vi "LabVIEW Task Manager.vi"() -> ()   [LabVIEW 2013, in "LVTM.lvlib"]
doc: "A debugging tool for use during LabVIEW development. Displays detailed information on all VIs in memory, belonging to a selected project/target. Allows for interacting with single or multiple selected VIs at a time; such as Open/Close their FP or BD, toggle execution highlighting, Pause/Resume/TogglePause their execution state, and more. Aborting selected VIs is also available for top-level VIs, but not for statically called SubVIs [reserved, waiting to run], nor most clones).\n\nNote: \"Refresh\" is not the same as \"Update\". The Update Speed determines how often State, Paused?, Hilite?, and Data Size properties are updated, plus removes items that are no longer in memory. A Refresh operation will repopulate the table with items which have come into memory since the last Refresh operation. A Refresh operation can be manually invoked from the View menu or by pressing F5, and is automatically invoked when any of the item Filter (include/exclude) options are toggled."
uses:
  LVTM.lvlib
  Controls_LVTM/View.ctl
  Controls_LVTM/SharedDataDVR.ctl
  Plugin/LVTM_Plugin.lvclass
  Controls_LVTM/LVTM_Config_Info.ctl
  TCP_Server/TCP_Server.lvclass
  <vilib>/GPower/Error/SubVIs/Filter/Error_FilterMulti.vi
  VIs_LVTM/FindName Task_Manager Library/FindName Task_Manager.lvlib
  DiscoverCommonTypeDefCallers.lvlib
  <userlib>/_SmartBalloon/Engine/Engine.lvclass
  HelpAbout_rha/RHA.lvlib
panel:
  in  "Search Clones Up To":i32=100 caption="Max Clones" min=0 step=1
  in  "Toggle Pause":bool
  in  "Pause":bool
  in  "Resume":bool
  in  "Do Not Highlight Execution":bool
  in  "Highlight Execution":bool
  in  "Close Front Panel":bool
  in  "Close Block Diagram":bool
  in  "Open Front Panel":bool
  in  "Open Block Diagram":bool
  in  "Abort":bool
  in  "App Instance:":u16(ring) items=["Default Application Instance", "Task Manager.lvproj:My Computer"]
  in  "View":T1
  out "NameFilterIsActive":bool
  out "FindIsActive":bool
  in  "error in":errorcluster
  in  "Refresh":bool
  in  "Data Tree":string[](tree)=["Get File Extension.vi"]
  out "Active Filters":string
  in  "Pause Source":string
  in  "Initialize":bool
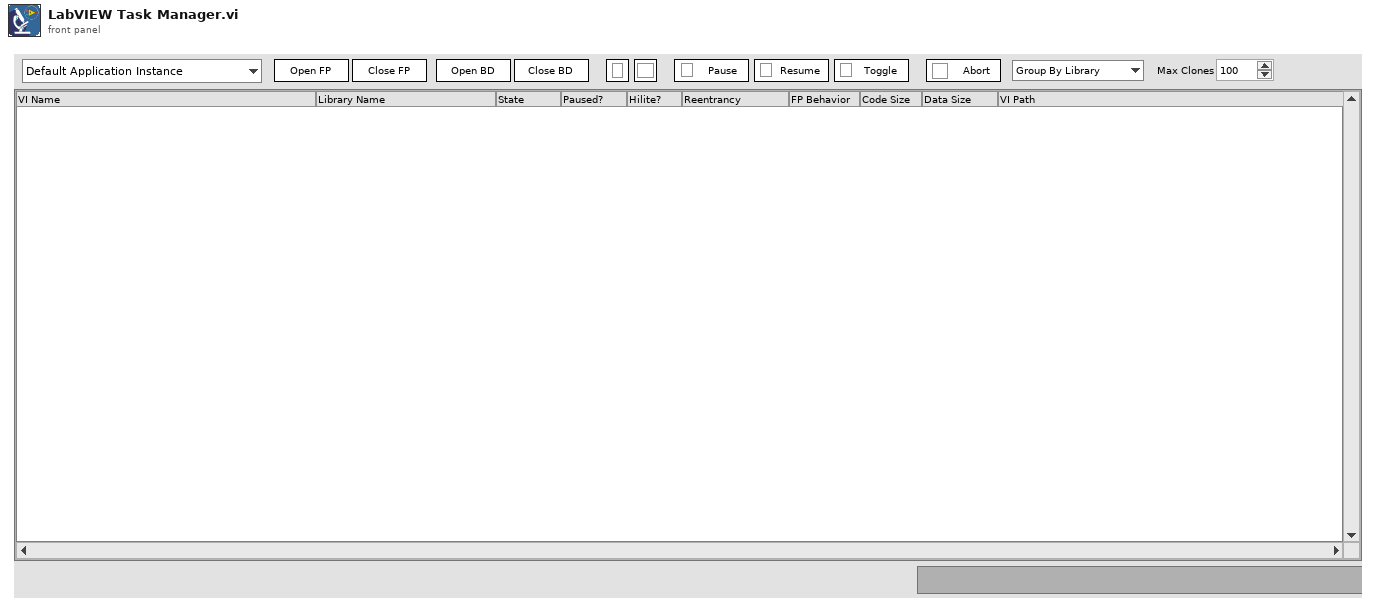
[diagram p1: front panel]
types:
  T1 = typedef "LVTM.lvlib/View.ctl" = enum16{"Group By Library", "Group By Folder", "Flat List"}
  T2 = typedef "LVTM.lvlib/LVTM_Config_Info.ctl" = cluster{"Data Tree Ref":refnum<vi>, "FP Ref":refnum<vi>, "Column Data Type":enum16{"String", "Numeric"}[], "Search Clones Up To":i32, "SortOptions":cluster{"Col.pri":i32, "RevDir.pri":bool, "Col.sec":i32, "RevDir.sec":bool}, "Group/Flat (0:group)":bool, "CollapsedNodes":string[], "Show/Hide Cols":bool[], "Filtered Paths":path[], "View":T1, "File Extension Filters":string[], "Filter Global VIs":bool, "Shared":refnum<data-value>, "Active Filters":refnum<vi>, "Refresh Rate (ms)":i32}
  T3 = cluster{"Shared":refnum<data-value>, "Plugins":refnum<class "LVTM_Plugin.lvclass">[], "UIConfig":T2}
  T4 = typedef "LVTM.lvlib/RequestEvents.ctl" = cluster{"Pause":refnum<user-event>, "Handle Error":refnum<user-event>, "Update Items":refnum<user-event>}
  T5 = typedef "LVTM.lvlib/SharedDataDVR.ctl" = cluster{"App":refnum<vi>, "VIs":string[]}
  T6 = enum16{"Share clones between instances", "Preallocate clone for each instance"}
  T7 = enum32{"Bad", "Idle", "Run top level", "Running"}
  T8 = typedef "LVPoint32TypeDef.ctl" = cluster{"Horizontal":i32, "Vertical":i32}
  T9 = enum32{"Invalid", "Standard", "Closed", "Hidden", "Minimized", "Maximized"}
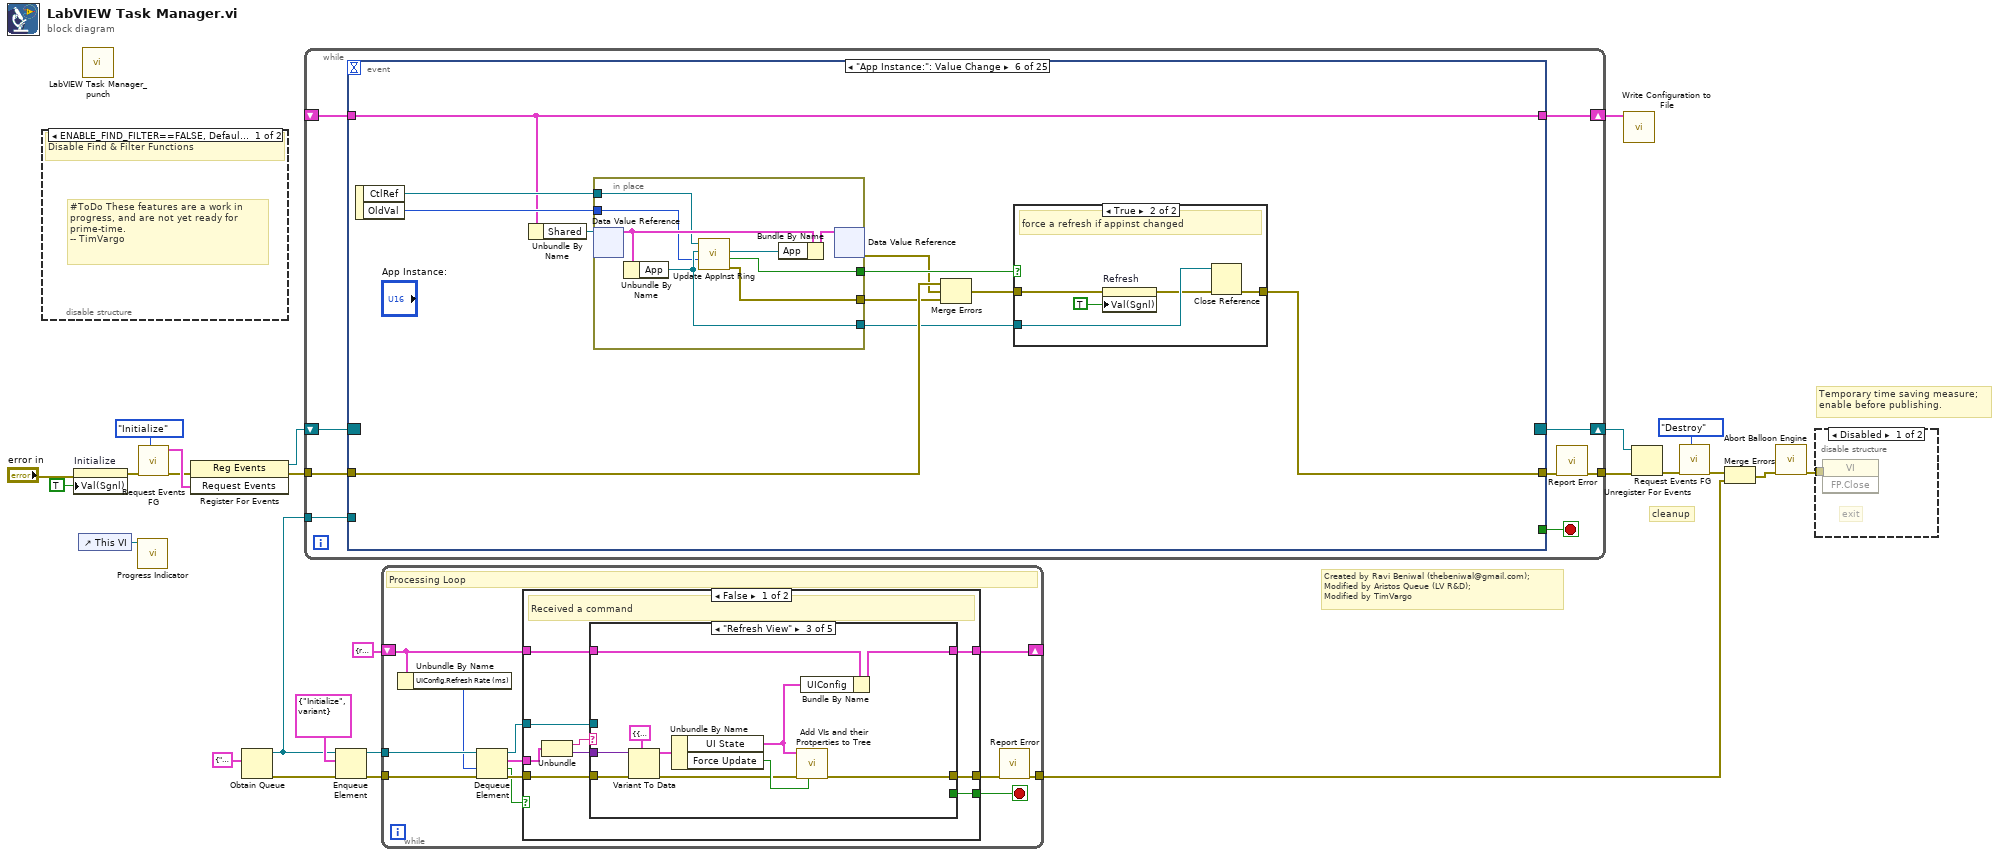
[diagram p0: block diagram]
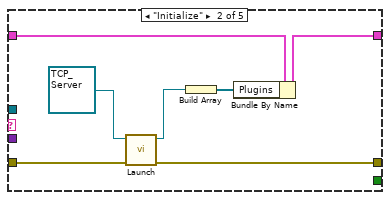
[diagram p4: hidden frame]
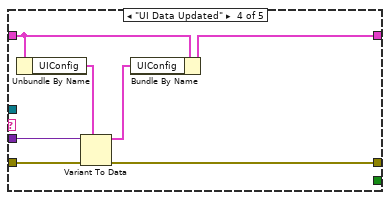
[diagram p5: hidden frame]
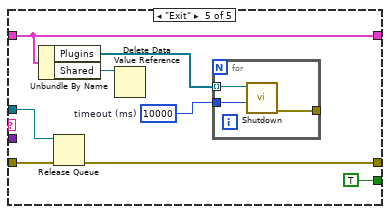
[diagram p6: hidden frame]
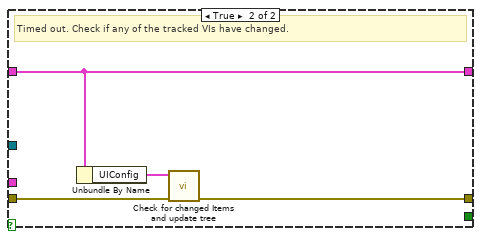
[diagram p7: hidden frame]
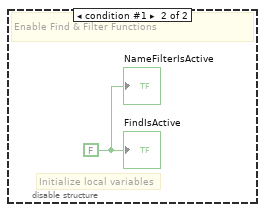
[diagram p8: hidden frame]
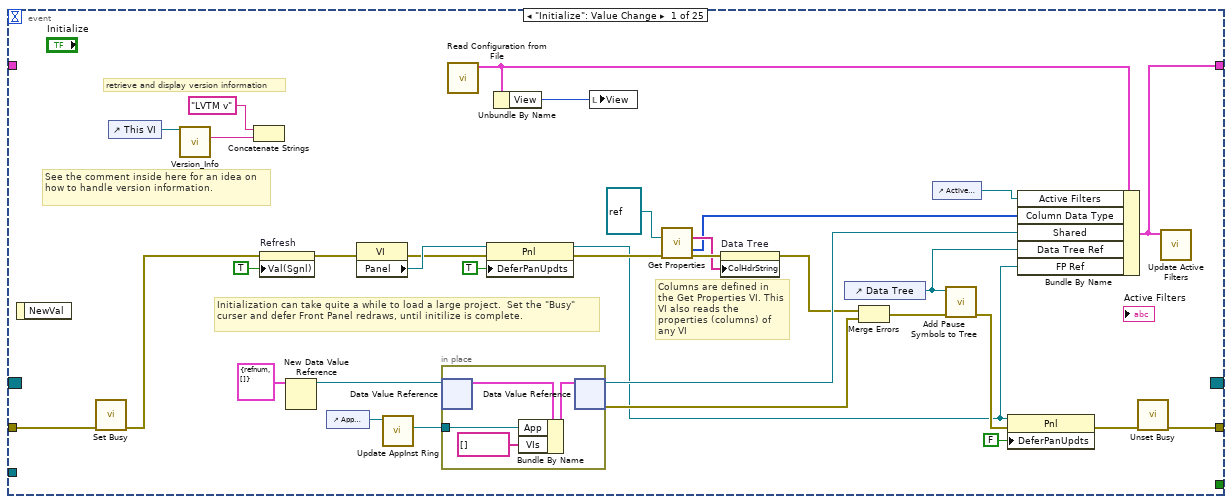
[diagram p9: hidden frame]
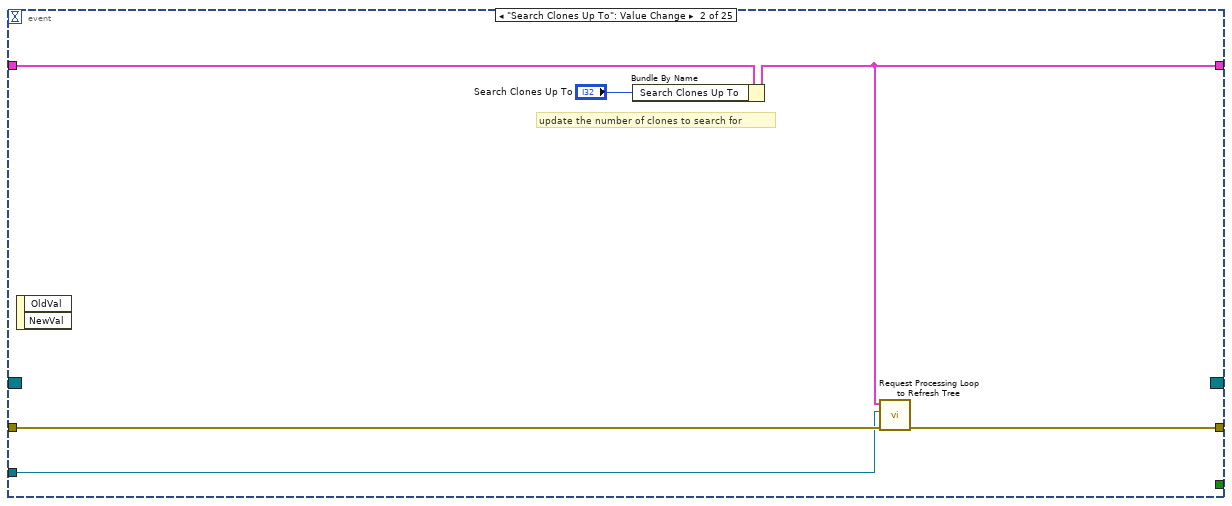
[diagram p10: hidden frame]
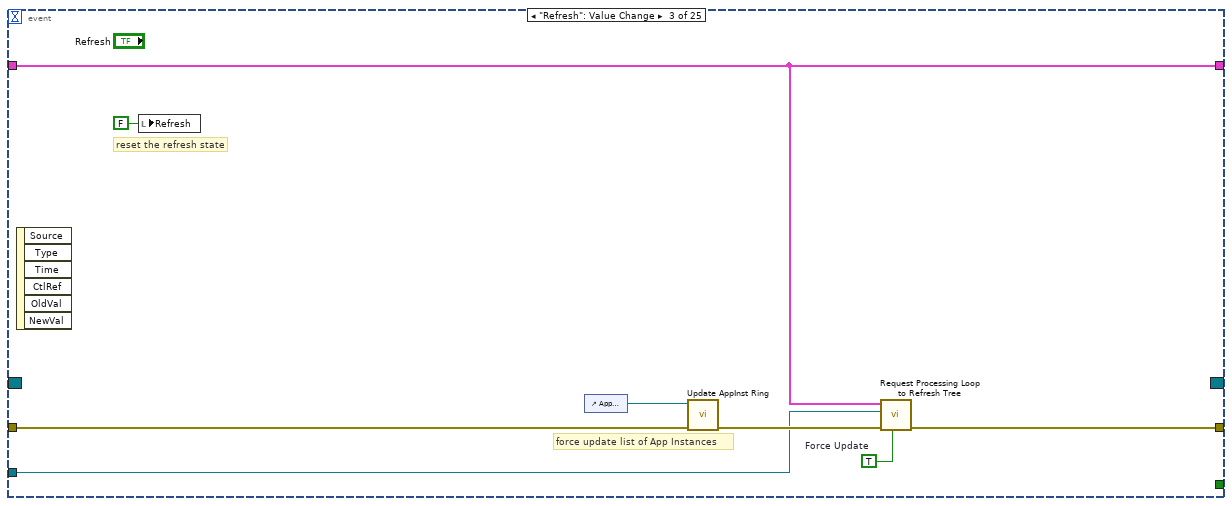
[diagram p11: hidden frame]
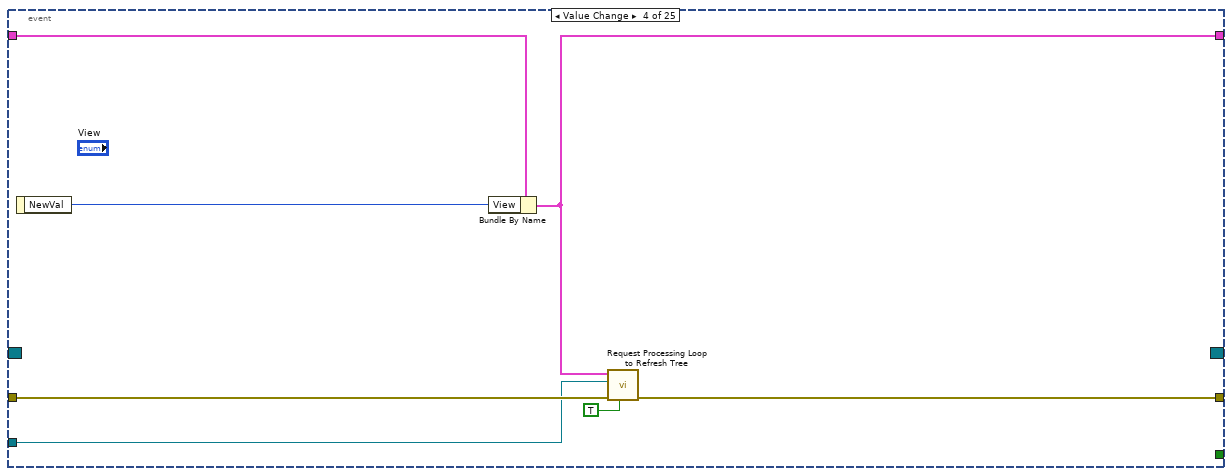
[diagram p12: hidden frame]
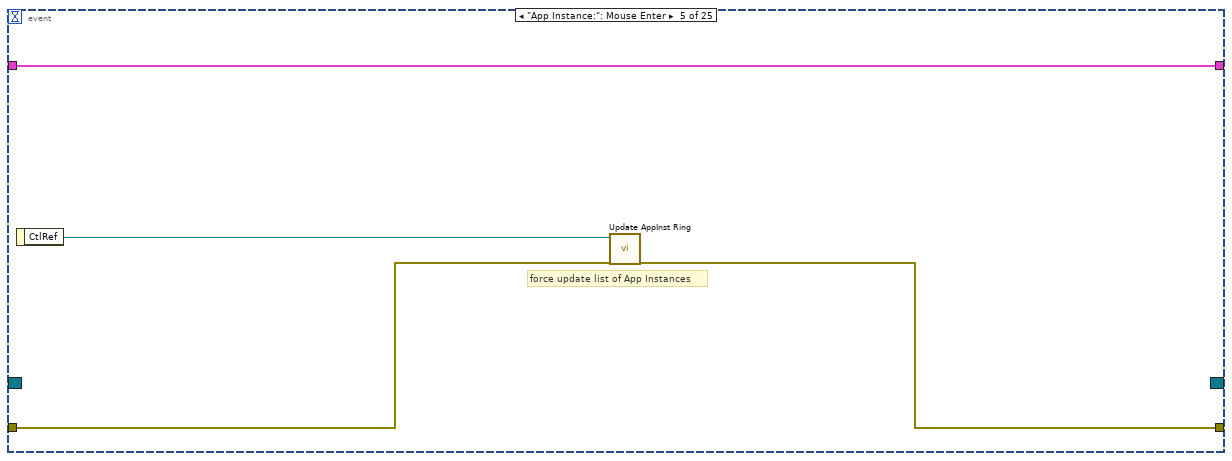
[diagram p13: hidden frame]
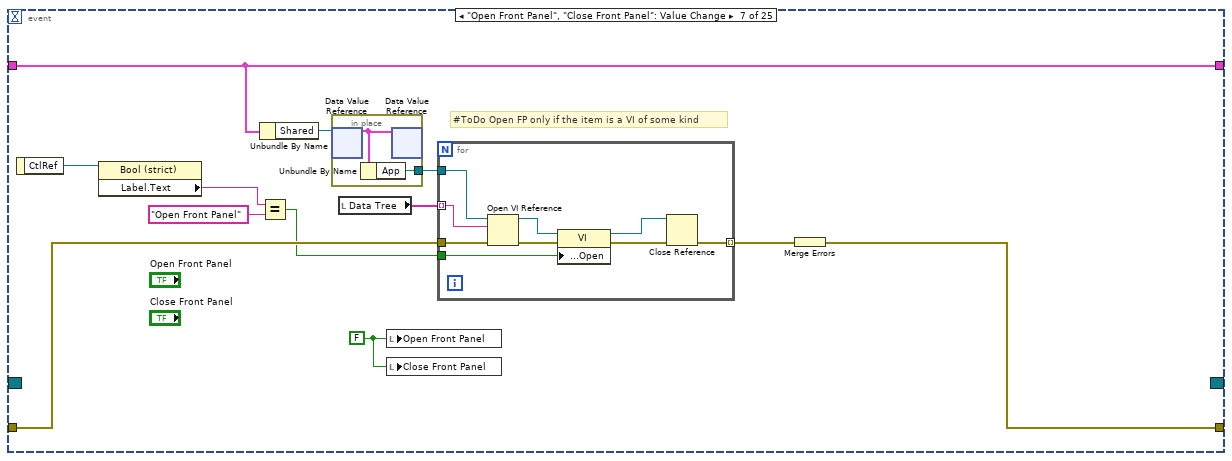
[diagram p15: hidden frame]
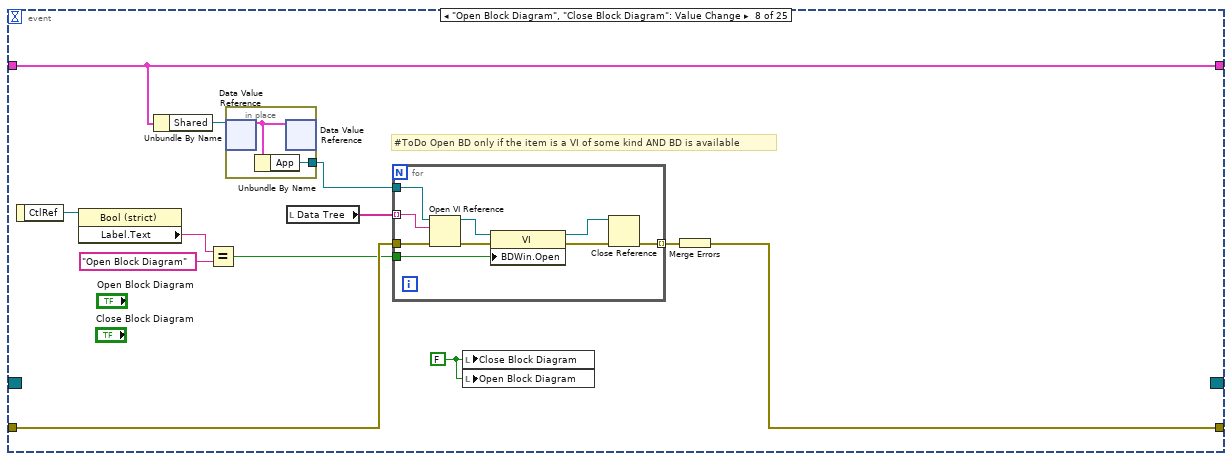
[diagram p16: hidden frame]
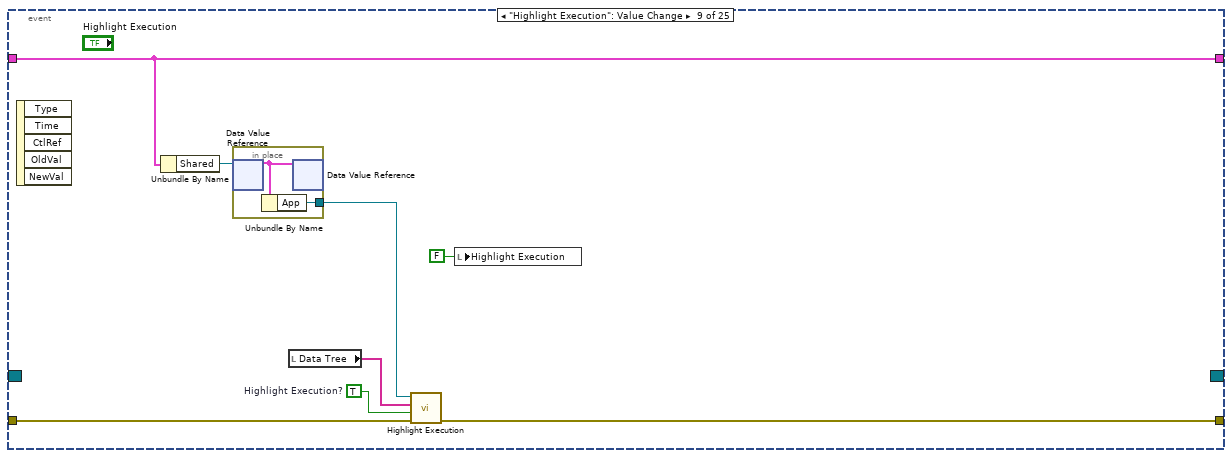
[diagram p17: hidden frame]
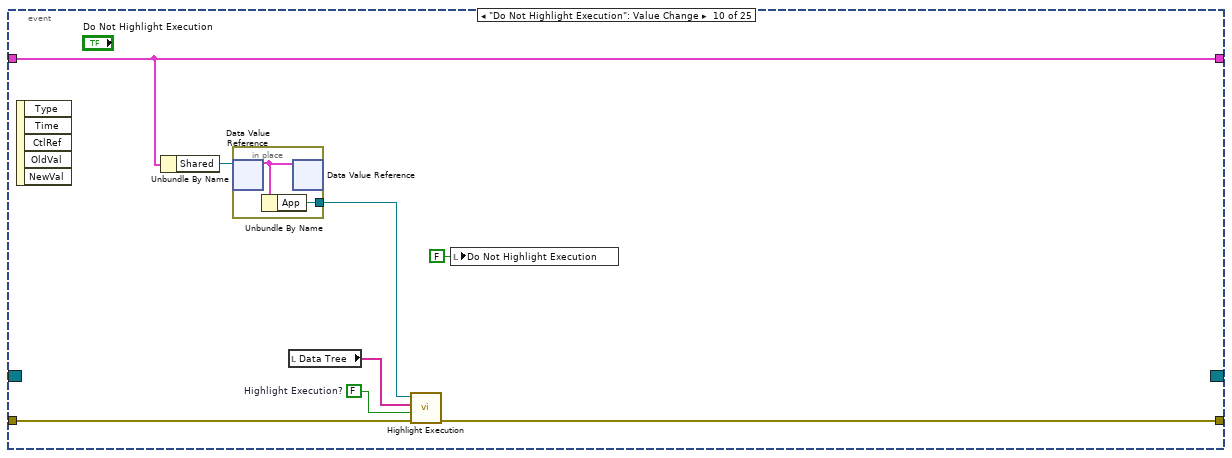
[diagram p18: hidden frame]
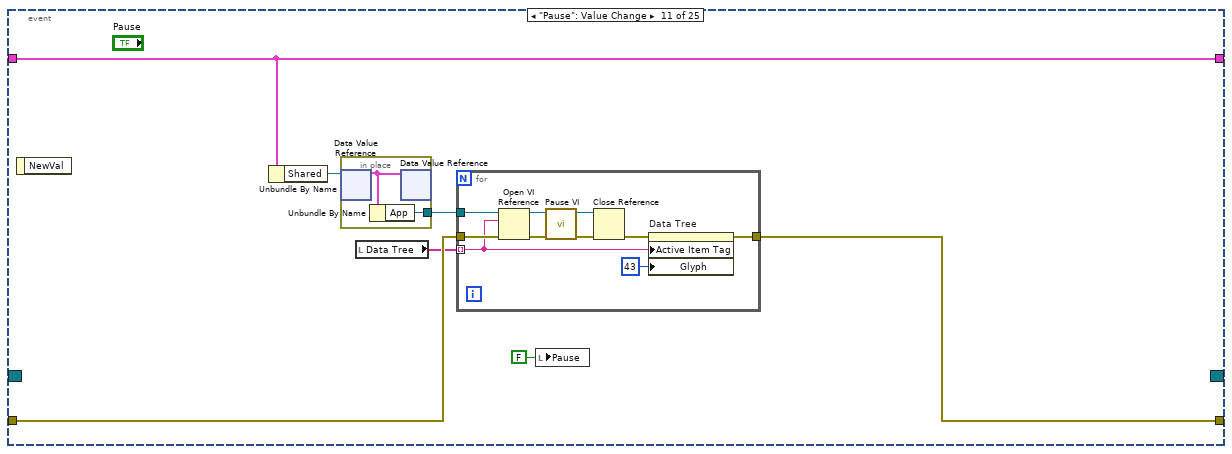
[diagram p19: hidden frame]
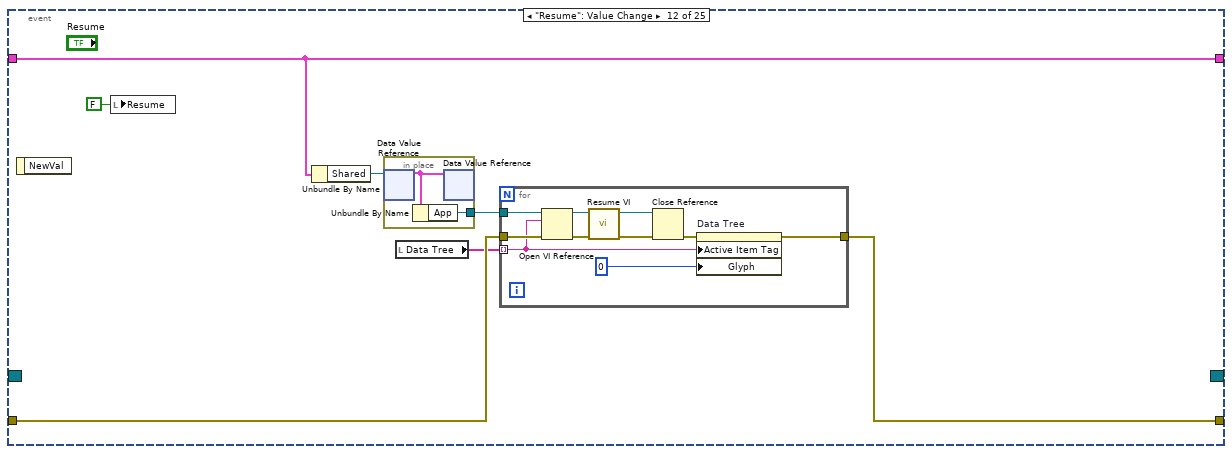
[diagram p20: hidden frame]
diagram:
  # "Temporary time saving measure;\nenable before publishing."
  # "cleanup"
  # "Created by Ravi Beniwal (thebeniwal@gmail.com);\nModified by Aristos Queue (LV R&D);\nModified by TimVargo"
  n1 = disable-structure shown="ENABLE_FIND_FILTER==FALSE, Default" {
    frame condition #0 (active) {
      # "#ToDo These features are a work in progress, and are not yet ready for prime-time.\n-- TimVargo"
      # "Disable Find & Filter Functions"
    }
    frame condition #1 {
      w26 = FALSE ("FindIsActive")
      # "Initialize local variables"
      # "Enable Find & Filter Functions"
      "FindIsActive" <- w26
      "NameFilterIsActive" <- w26
    }
  }
  n2 = property on="Initialize" class="Bool (strict)"(error in="error in", "Val(Sgnl)"=TRUE ("Value (Signaling)")) -> (error out=w16:errorcluster)  [unwired: 1 in, 1 out]
  n3 = control-ref of="This VI"() -> (w9:refnum<vi>)
  n4 = call "LabVIEW Task Manager_punch.vi"() -> ()  [unwired: 12 in]
  n5 = call "Progress Indicator.vi"("Main VI Ref"=w9) -> ()  [unwired: 11 in]
  n6 = call "Request Events FG.vi"("Action (Get)"=enum16{"Initialize", "Get", "Destroy"}."Initialize" ("Action"), "error in"=w16) -> ("error out"=w15:errorcluster, "Request Events"=w18:T4)  [unwired: 8 in]
  n7 = register-events(error in=w15, w18) -> (reference out=w23:refnum<event-registration>, error out=w22:errorcluster)  [unwired: 1 in]
  n8 = Obtain Queue(element data type=cluster{"Command":string, "Data":variant} {"Command"="", "Data"=variant}) -> (queue out=w7:refnum<queue>, error out=w5:errorcluster)  [unwired: 4 in, 1 out]
  n9 = while {
    shift-right: [w27] -> w10
    shift-left: _ -> [w34]
    shift-right: [w33] -> w24
    shift-left: w23 -> [w32]
    tunnel: w22 -> [w31]
    tunnel: [w29] -> w21
    tunnel: w7 -> [w28]
    stop <- w35 stop-if-true
    n10 = event shown="[5] \"App Instance:\": Value Change" {
      selector: w32 -> [_ _ _ _ _ _ _ _ _ _ _ _ _ _ _ _ _ _ _ _ _ _ _ _ _]
      dyn-events: [_ _ _ _ _ _ _ _ _ _ _ _ _ _ _ _ _ _ _ _ _ _ _ _ _] -> w33
      timeout: _ -> [_ _ _ _ _ _ _ _ _ _ _ _ _ _ _ _ _ _ _ _ _ _ _ _ _]
      tunnel: [_ _ _ _ _ _ _ _ _ _ _ _ _ _ _ _ _ _ w457 TRUE ("stop") _ _ w519 _ _] -> w35
      tunnel: w34 -> [_ w78 w85 w93 w97 w101 w125 w148 w172 w182 w195 w209 w231 w253 w294 w301 w357 w397 w464 w470 w481 w483 w515 w718 w751]
      tunnel: [w38 w74 w85 w88 w97 w101 w125 w148 w172 w182 w195 w209 w231 w253 w294 w302 w357 w397 w464 w470 w481 w483 w514 w718 w749] -> w27
      tunnel: w31 -> [w61 w77 w84 w92 w95 w108 w134 w157 w176 w186 w194 w214 w228 w256 w291 w300 w364 w402 w456 w472 _ w492 w517 w719 w752]
      tunnel: [w59 w76 w82 w91 w94 w107 w127 w150 w175 w185 w193 w213 w230 w255 w290 w296 w362 w401 w456 w469 _ w487 w516 w717 w750] -> w30
      tunnel: w28 -> [_ w73 w81 w87 _ _ _ _ _ _ _ _ _ _ _ w295 _ _ w455 w471 _ _ w513 _ _]
      event "Initialize": Value Change {
        # "See the comment inside here for an idea on how to handle version information."
        # "retrieve and display version information"
        # "Initialization can take quite a while to load a large project.  Set the \"Busy\" curser and defer Front Panel redraws, until initilize is complete."
        # "Columns are defined in the Get Properties VI. This VI also reads the properties (columns) of any VI"
        n11 = event-data() -> ()  [unwired: 2 out]
        n12 = call <vilib>:"Set Busy.vi"("error in (no error)"=w61) -> ("error out"=w54:errorcluster)  [unwired: 9 in, 1 out]
        n13 = control-ref of="This VI"() -> (w50:refnum<vi>)
        n14 = call "Version_Info.vi"("Generic VI Reference"=w50) -> ("FileVersion_Str"=w49:string)  [unwired: 8 in, 2 out]
        n15 = Concatenate Strings("LVTM v" ("string"), w49) -> ()  [unwired: 1 out]
        n16 = property on="Refresh" class="Bool (strict)"(error in=w54, "Val(Sgnl)"=TRUE ("Value (Signaling)")) -> (error out=w66:errorcluster)  [unwired: 1 in, 1 out]
        n17 = New Data Value Reference(data value=T5 {"App"=refnum, "VIs"=[]}) -> (data value reference=w36:refnum<data-value>)  [unwired: 1 in, 1 out]
        n18 = control-ref of="App Instance:"() -> (w67:refnum<vi>)
        n19 = property class="VI"(error in=w66) -> (error out=w52:errorcluster, "Panel"=w53:refnum<vi>)  [unwired: 1 in, 1 out]
        n20 = call "Update AppInst Ring.vi"("Ring in"=w67) -> ("AppInst out"=w47:refnum<vi>)  [unwired: 8 in, 2 out]
        n21 = in-place {
          in-place-border: w47 -> [w69]
          n22 = in-place-dvr #1(w36) -> (w72:T5)  [unwired: 1 out]
          n23 = Bundle By Name(cluster=w72, "App"=w69, "VIs"=string[] []) -> (w71:T5)
          n24 = in-place-dvr #1(w71) -> (w46:refnum<data-value>, w43:errorcluster)
        }
        n25 = call "Read Configuration from File.vi"() -> ("Configuration"=w41:T2)  [unwired: 10 in, 1 out]
        n26 = property class="Pnl"(reference=w53, error in=w52, "DeferPanUpdts"=TRUE ("Defer Panel Updates")) -> (reference out=w40:refnum<vi>, error out=w51:errorcluster)
        n27 = Unbundle By Name(w41) -> ("View"=w42:T1)
        n28 = local write "View"(w42) -> ()
        n29 = call "Get Properties.vi"("AppInst"=refnum<vi> refnum, "error in"=w51) -> ("Column Labels"=w64:string[], "Column Data Type"=w60:enum16{"String", "Numeric"}[], "error out"=w65:errorcluster)  [unwired: 4 in, 7 out]
        n30 = property on="Data Tree" class="Tree (strict)"(error in=w65, "ColHdrString"=w64) -> (error out=w45:errorcluster)  [unwired: 1 in, 1 out]
        n31 = control-ref of="Data Tree"() -> (w62:refnum<vi>)
        n32 = Merge Errors(w45, w43) -> (w44:errorcluster)
        n33 = control-ref of="Active Filters"() -> (w39:refnum<vi>)
        n34 = call "Add Pause Symbols to Tree.vi"("error in"=w44, "Data Tree Ref"=w62) -> ("error out"=w56:errorcluster)  [unwired: 9 in]
        n35 = property class="Pnl"(reference=w40, error in=w56, "DeferPanUpdts"=FALSE ("Defer Panel Updates")) -> (error out=w55:errorcluster)  [unwired: 1 out]
        n36 = Bundle By Name(cluster=w41, "Active Filters"=w39, "Column Data Type"=w60, "Shared"=w46, "Data Tree Ref"=w62, "FP Ref"=w40) -> (w38:T2)
        n37 = call <vilib>:"Unset Busy.vi"("error in (no error)"=w55) -> ("error out"=w59:errorcluster)  [unwired: 10 in]
        n38 = call "Update Active Filters.vi"("Configuration"=w38) -> ()  [unwired: 10 in, 1 out]
      }
      event "Search Clones Up To": Value Change {
        # "update the number of clones to search for"
        n39 = event-data() -> ()  [unwired: 3 out]
        n40 = Bundle By Name(cluster=w78, "Search Clones Up To"="Search Clones Up To") -> (w74:T2)
        n41 = call "Request Processing Loop to Refresh Tree.vi"("error in (no error)"=w77, "Queue in"=w73, "ConfigInfo in"=w74) -> ("error out"=w76:errorcluster)  [unwired: 8 in]
      }
      event "Refresh": Value Change {
        w79 = TRUE  # Force Update
        # "reset the refresh state"
        # "force update list of App Instances"
        n42 = event-data() -> ()  [unwired: 7 out]
        n43 = local write "Refresh"(FALSE ("Refresh")) -> ()
        n44 = control-ref of="App Instance:"() -> (w86:refnum<vi>)
        n45 = call "Update AppInst Ring.vi"("error in"=w84, "Ring in"=w86) -> ("error out"=w83:errorcluster)  [unwired: 7 in, 2 out]
        n46 = call "Request Processing Loop to Refresh Tree.vi"("Force Update"=w79, "error in (no error)"=w83, "Queue in"=w81, "ConfigInfo in"=w85) -> ("error out"=w82:errorcluster)  [unwired: 7 in]
      }
      event Value Change {
        n47 = event-data() -> ("NewVal"=w90:T1)  [unwired: 1 out]
        n48 = Bundle By Name(cluster=w93, "View"=w90) -> (w88:T2)
        n49 = call "Request Processing Loop to Refresh Tree.vi"("Force Update"=TRUE ("Force Tree Update (F)"), "error in (no error)"=w92, "Queue in"=w87, "ConfigInfo in"=w88) -> ("error out"=w91:errorcluster)  [unwired: 7 in]
      }
      event "App Instance:": Mouse Enter {
        # "force update list of App Instances"
        n50 = event-data() -> ("CtlRef"=w96:refnum<vi>)  [unwired: 1 out]
        n51 = call "Update AppInst Ring.vi"("error in"=w95, "Ring in"=w96) -> ("error out"=w94:errorcluster)  [unwired: 7 in, 2 out]
      }
      event "App Instance:": Value Change {
        n52 = event-data() -> ("CtlRef"=w104:refnum<vi>, "OldVal"=w103:u16)  [unwired: 1 out]
        n53 = Unbundle By Name(w101) -> ("Shared"=w106:refnum<data-value>)
        n54 = in-place {
          in-place-border: [w114] -> w105
          in-place-border: w104 -> [w115]
          in-place-border: w103 -> [w113]
          in-place-border: [w110] -> w102
          in-place-border: [w109] -> w98
          n55 = in-place-dvr #2(w106) -> (w116:T5)  [unwired: 1 out]
          n56 = Unbundle By Name(w116) -> ("App"=w114:refnum<vi>)
          n57 = call "Update AppInst Ring.vi"("Old Value"=w113, "AppInst in"=w114, "Ring in"=w115) -> ("error out"=w109:errorcluster, "Selection Changed?"=w110:bool, "AppInst out"=w111:refnum<vi>)  [unwired: 6 in]
          n58 = Bundle By Name(cluster=w116, "App"=w111) -> (w112:T5)
          n59 = in-place-dvr #2(w112) -> (w99:errorcluster)  [unwired: 1 out]
        }
        n60 = Merge Errors(w108, w99, w98) -> (w100:errorcluster)
        n61 = case shown="True" w102 {
          tunnel: w105 -> [_ w121]
          tunnel: w100 -> [w117 w120]
          tunnel: [w117 w118] -> w107
          frame False {
            # "do nothing"
          }
          frame True {
            # "force a refresh if appinst changed"
            n62 = property on="Refresh" class="Bool (strict)"(error in=w120, "Val(Sgnl)"=TRUE ("Value (Signaling)")) -> (error out=w119:errorcluster)  [unwired: 1 in, 1 out]
            n63 = Close Reference(reference=w121, error in (no error)=w119) -> (error out=w118:errorcluster)
          }
        }
      }
      event "Open Front Panel", "Close Front Panel": Value Change {
        w123 = FALSE ("Open Front Panel")
        # "#ToDo Open FP only if the item is a VI of some kind"
        n64 = event-data() -> ("CtlRef"=w131:refnum<vi>)  [unwired: 1 out]
        n65 = property class="Bool (strict)"(reference=w131) -> ("Label.Text"=w129:string)  [unwired: 1 in, 2 out]
        n66 = Unbundle By Name(w125) -> ("Shared"=w126:refnum<data-value>)
        n67 = Equal?(x=w129, y="Open Front Panel") -> (x = y?=w128:bool)
        n68 = in-place {
          in-place-border: [w135] -> w124
          n69 = in-place-dvr #3(w126) -> (w136:T5)  [unwired: 1 out]
          n70 = Unbundle By Name(w136) -> ("App"=w135:refnum<vi>)
          n71 = in-place-dvr #3(w136) -> ()  [unwired: 2 out]
        }
        n72 = local read "Data Tree"() -> (w132:string[])
        n73 = local write "Open Front Panel"(w123) -> ()
        n74 = local write "Close Front Panel"(w123) -> ()
        n75 = for {
          tunnel: [w145] -> w133 mode=indexing
          tunnel: w134 -> [w144]
          tunnel: w132 -> [w143] mode=indexing
          tunnel: w124 -> [w138]
          tunnel: w128 -> [w137]
          n76 = Open VI Reference(application reference (local)=w138, vi path=w143, error in (no error)=w144) -> (vi reference=w141:refnum<vi>, error out=w142:errorcluster)  [unwired: 3 out]
          n77 = property class="VI"(reference=w141, error in=w142, "Front Panel.Open"=w137) -> (reference out=w140:refnum<vi>, error out=w139:errorcluster)
          n78 = Close Reference(reference=w140, error in (no error)=w139) -> (error out=w145:errorcluster)
        }
        n79 = Merge Errors(w133) -> (w127:errorcluster)
      }
      event "Open Block Diagram", "Close Block Diagram": Value Change {
        w146 = FALSE ("Close Block Diagram")
        # "#ToDo Open BD only if the item is a VI of some kind AND BD is available"
        n80 = event-data() -> ("CtlRef"=w152:refnum<vi>)  [unwired: 1 out]
        n81 = property class="Bool (strict)"(reference=w152) -> ("Label.Text"=w153:string)  [unwired: 1 in, 2 out]
        n82 = Unbundle By Name(w148) -> ("Shared"=w149:refnum<data-value>)
        n83 = Equal?(x=w153, y="Open Block Diagram") -> (x = y?=w151:bool)
        n84 = in-place {
          in-place-border: [w158] -> w147
          n85 = in-place-dvr #4(w149) -> (w159:T5)  [unwired: 1 out]
          n86 = Unbundle By Name(w159) -> ("App"=w158:refnum<vi>)
          n87 = in-place-dvr #4(w159) -> ()  [unwired: 2 out]
        }
        n88 = local read "Data Tree"() -> (w155:string[])
        n89 = for {
          tunnel: [w168] -> w156 mode=indexing
          tunnel: w157 -> [w167]
          tunnel: w155 -> [w166] mode=indexing
          tunnel: w147 -> [w161]
          tunnel: w151 -> [w160]
          n90 = Open VI Reference(application reference (local)=w161, vi path=w166, error in (no error)=w167) -> (vi reference=w164:refnum<vi>, error out=w165:errorcluster)  [unwired: 3 out]
          n91 = property class="VI"(reference=w164, error in=w165, "BDWin.Open"=w160) -> (reference out=w163:refnum<vi>, error out=w162:errorcluster)
          n92 = Close Reference(reference=w163, error in (no error)=w162) -> (error out=w168:errorcluster)
        }
        n93 = local write "Close Block Diagram"(w146) -> ()
        n94 = local write "Open Block Diagram"(w146) -> ()
        n95 = Merge Errors(w156) -> (w150:errorcluster)
      }
      event "Highlight Execution": Value Change {
        w169 = TRUE  # Highlight Execution?
        n96 = event-data() -> ()  [unwired: 6 out]
        n97 = Unbundle By Name(w172) -> ("Shared"=w173:refnum<data-value>)
        n98 = in-place {
          in-place-border: [w177] -> w171
          n99 = in-place-dvr #5(w173) -> (w178:T5)  [unwired: 1 out]
          n100 = Unbundle By Name(w178) -> ("App"=w177:refnum<vi>)
          n101 = in-place-dvr #5(w178) -> ()  [unwired: 2 out]
        }
        n102 = local read "Data Tree"() -> (w174:string[])
        n103 = call "Highlight Execution.vi"("error in (no error)"=w176, "Highlight Execution?"=w169, "VIs"=w174, "Application in"=w171) -> ("error out"=w175:errorcluster)  [unwired: 7 in]
        n104 = local write "Highlight Execution"(FALSE ("Toggle ExecHilite")) -> ()
      }
      event "Do Not Highlight Execution": Value Change {
        w179 = FALSE  # Highlight Execution?
        n105 = event-data() -> ()  [unwired: 6 out]
        n106 = Unbundle By Name(w182) -> ("Shared"=w183:refnum<data-value>)
        n107 = in-place {
          in-place-border: [w187] -> w181
          n108 = in-place-dvr #6(w183) -> (w188:T5)  [unwired: 1 out]
          n109 = Unbundle By Name(w188) -> ("App"=w187:refnum<vi>)
          n110 = in-place-dvr #6(w188) -> ()  [unwired: 2 out]
        }
        n111 = local read "Data Tree"() -> (w184:string[])
        n112 = call "Highlight Execution.vi"("error in (no error)"=w186, "Highlight Execution?"=w179, "VIs"=w184, "Application in"=w181) -> ("error out"=w185:errorcluster)  [unwired: 7 in]
        n113 = local write "Do Not Highlight Execution"(FALSE ("Toggle ExecHilite")) -> ()
      }
      event "Pause": Value Change {
        n114 = event-data() -> ()  [unwired: 2 out]
        n115 = Unbundle By Name(w195) -> ("Shared"=w191:refnum<data-value>)
        n116 = in-place {
          in-place-border: [w196] -> w190
          n117 = in-place-dvr #7(w191) -> (w197:T5)  [unwired: 1 out]
          n118 = Unbundle By Name(w197) -> ("App"=w196:refnum<vi>)
          n119 = in-place-dvr #7(w197) -> ()  [unwired: 2 out]
        }
        n120 = local read "Data Tree"() -> (w192:string[])
        n121 = for {
          tunnel: w192 -> [w200] mode=indexing
          tunnel: w194 -> [w203]
          tunnel: [w201] -> w193
          tunnel: w190 -> [w198]
          n122 = Open VI Reference(application reference (local)=w198, vi path=w200, error in (no error)=w203) -> (vi reference=w206:refnum<vi>, error out=w207:errorcluster)  [unwired: 3 out]
          n123 = call "Pause VI.vi"("error in (no error)"=w207, "VI in"=w206) -> ("error out"=w204:errorcluster, "VI out"=w205:refnum<vi>)  [unwired: 8 in]
          n124 = Close Reference(reference=w205, error in (no error)=w204) -> (error out=w202:errorcluster)
          n125 = property on="Data Tree" class="Tree (strict)"(error in=w202, "Active Item Tag"=w200, "Glyph"=43 ("Active Item:Symbol Index")) -> (error out=w201:errorcluster)  [unwired: 1 in, 1 out]
        }
        n126 = local write "Pause"(FALSE ("Pause")) -> ()
      }
      event "Resume": Value Change {
        n127 = event-data() -> ()  [unwired: 2 out]
        n128 = local write "Resume"(FALSE ("Resume")) -> ()
        n129 = Unbundle By Name(w209) -> ("Shared"=w210:refnum<data-value>)
        n130 = in-place {
          in-place-border: [w215] -> w208
          n131 = in-place-dvr #8(w210) -> (w216:T5)  [unwired: 1 out]
          n132 = Unbundle By Name(w216) -> ("App"=w215:refnum<vi>)
          n133 = in-place-dvr #8(w216) -> ()  [unwired: 2 out]
        }
        n134 = local read "Data Tree"() -> (w212:string[])
        n135 = for {
          tunnel: w212 -> [w218] mode=indexing
          tunnel: w214 -> [w222]
          tunnel: [w219] -> w213
          tunnel: w208 -> [w217]
          n136 = Open VI Reference(application reference (local)=w217, vi path=w218, error in (no error)=w222) -> (vi reference=w225:refnum<vi>, error out=w226:errorcluster)  [unwired: 3 out]
          n137 = call "Resume VI.vi"("error in (no error)"=w226, "VI in"=w225) -> ("error out"=w223:errorcluster, "VI out"=w224:refnum<vi>)  [unwired: 8 in]
          n138 = Close Reference(reference=w224, error in (no error)=w223) -> (error out=w220:errorcluster)
          n139 = property on="Data Tree" class="Tree (strict)"(error in=w220, "Active Item Tag"=w218, "Glyph"=0 ("Active Item:Symbol Index")) -> (error out=w219:errorcluster)  [unwired: 1 in, 1 out]
        }
      }
      event "Toggle Pause": Value Change {
        n140 = event-data() -> ()  [unwired: 2 out]
        n141 = local write "Toggle Pause"(FALSE ("Resume")) -> ()
        n142 = Unbundle By Name(w231) -> ("Shared"=w232:refnum<data-value>)
        n143 = in-place {
          in-place-border: [w249] -> w229
          n144 = in-place-dvr #9(w232) -> (w250:T5)  [unwired: 1 out]
          n145 = Unbundle By Name(w250) -> ("App"=w249:refnum<vi>)
          n146 = in-place-dvr #9(w250) -> ()  [unwired: 2 out]
        }
        n147 = local read "Data Tree"() -> (w227:string[])
        n148 = for {
          tunnel: w227 -> [w245] mode=indexing
          tunnel: w228 -> [w248]
          tunnel: [w246] -> w230
          tunnel: w229 -> [w244]
          # "Despite the method name, this\ntoggles Pause/Resume."
          n149 = Open VI Reference(application reference (local)=w244, vi path=w245, error in (no error)=w248) -> (vi reference=w242:refnum<vi>, error out=w243:errorcluster)  [unwired: 3 out]
          n150 = invoke class="VI" method="PauseVI"(reference=w242, error in=w243) -> (reference out=w241:refnum<vi>, error out=w240:errorcluster)  [unwired: 1 in, 1 out]
          n151 = property class="VI"(reference=w241, error in=w240) -> (reference out=w238:refnum<vi>, error out=w239:errorcluster, "Is VI Paused?"=w237:bool)
          n152 = Close Reference(reference=w238, error in (no error)=w239) -> (error out=w247:errorcluster)
          n153 = Select(t=43, s=w237, f=0 ("Active Item:Symbol Index")) -> (s? t:f=w234:i32)
          n154 = property on="Data Tree" class="Tree (strict)"(error in=w247, "Active Item Tag"=w245, "Glyph"=w234) -> (error out=w246:errorcluster)  [unwired: 1 in, 1 out]
        }
      }
      event "Abort": Value Change {
        # "Only VIs running at top level may be aborted."
        # "#ToDo this is where the string 'error' was being placed into the 'library name' column (left of the 'State' column).  This is fixed for now by changing hardwired column number from 1 to 2, but the column number will later need logic to calculate the correct column, once the flat (non-grouped) option is implemented, which will hide the 'library name' column."
        n155 = event-data() -> ()  [unwired: 2 out]
        n156 = Unbundle By Name(w253) -> ("Shared"=w254:refnum<data-value>)
        n157 = local write "Abort"(FALSE ("Abort")) -> ()
        n158 = in-place {
          in-place-border: [w258] -> w252
          n159 = in-place-dvr #10(w254) -> (w259:T5)  [unwired: 1 out]
          n160 = Unbundle By Name(w259) -> ("App"=w258:refnum<vi>)
          n161 = in-place-dvr #10(w259) -> ()  [unwired: 2 out]
        }
        n162 = for {
          tunnel: [w268] -> w255
          tunnel: "Data Tree" -> [w267] mode=indexing
          tunnel: w252 -> [w266]
          tunnel: w256 -> [w265]
          n163 = Open VI Reference(application reference (local)=w266, vi path=w267, error in (no error)=w265) -> (vi reference=w262:refnum<vi>, error out=w264:errorcluster)  [unwired: 3 out]
          n164 = property class="VI"(reference=w262, error in=w264) -> (reference out=w261:refnum<vi>, error out=w263:errorcluster, "Exec.State"=w260:T7)
          n165 = case shown="\"Run top level\"" w260 {
            tunnel: [w269 w281] -> w268
            tunnel: w267 -> [_ w279]
            tunnel: w263 -> [w271 w274]
            tunnel: w261 -> [w270 w273]
            frame "Bad", Default {
              n166 = Close Reference(reference=w270, error in (no error)=w271) -> (error out=w269:errorcluster)
            }
            frame "Run top level" {
              n167 = invoke class="VI" method="Abort VI"(reference=w273, error in=w274) -> (reference out=w283:refnum<vi>, error out=w275:errorcluster)  [unwired: 1 in, 1 out]
              n168 = property class="VI"(reference=w283, error in=w275) -> (reference out=w282:refnum<vi>, error out=w277:errorcluster, "Exec.State"=w284:T7)
              n169 = Close Reference(reference=w282, error in (no error)=w277) -> (error out=w272:errorcluster)
              n170 = case shown="No Error" w272 {
                selector: w272 -> [w285 _]
                tunnel: w284 -> [w288 _]
                tunnel: [w287 "Error"] -> w280
                tunnel: [w286 _] -> w276
                frame No Error {
                  n171 = Format Into String(error in=w285, w288) -> (resulting string=w287:string, error out=w286:errorcluster)  [unwired: 2 in]
                }
                frame Error {
                }
              }
              n172 = property on="Data Tree" class="Tree (strict)"(error in=w276, "Active Item Tag"=w279, "ActiveColNum"=2 ("Active Cell:Active Column Number"), "Cell String"=w280) -> (error out=w281:errorcluster)  [unwired: 1 in, 1 out]
            }
          }
        }
      }
      event "Pause Source": Value Change {
        n173 = event-data() -> ("NewVal"=w292:string)  [unwired: 1 out]
        n174 = property on="Data Tree" class="Tree (strict)"(error in=w291, "Active Item Tag"=w292, "Glyph"=44 ("Active Item:Symbol Index")) -> (error out=w290:errorcluster)  [unwired: 1 in, 1 out]
      }
      event "Data Tree": Mouse Down {
        n175 = event-data() -> ("Coords"=w303:T8)  [unwired: 1 out]
        n176 = invoke on="Data Tree" class="Tree (strict)" method="Point To Row Column"(error in=w300, "Point"=w303) -> (error out=w298:errorcluster, "Tag"=w299:string, "Col"=w297:i32)  [unwired: 6 in, 5 out]
        n177 = case shown="\"TREE_COLUMN_HEADERS\"" w299 {
          tunnel: w298 -> [w305 w322]
          tunnel: w297 -> [_ w325]
          tunnel: [w305 w317] -> w296
          tunnel: [w304 w308] -> w302
          tunnel: w301 -> [w304 w330]
          tunnel: w295 -> [_ w307]
          frame Default {
          }
          frame "TREE_COLUMN_HEADERS" {
            n178 = Unbundle By Name(w330) -> ("Data Tree Ref"=w313:refnum<vi>, "SortOptions.RevDir.pri"=w312:bool, "SortOptions.Col.pri"=w311:i32, "SortOptions.RevDir.sec"=w310:bool, "SortOptions.Col.sec"=w309:i32, "Column Data Type"=w326:enum16{"String", "Numeric"}[], "FP Ref"=w320:refnum<vi>)
            n179 = property class="Pnl"(reference=w320, error in=w322, "DeferPanUpdts"=TRUE ("Defer Panel Updates")) -> (reference out=w316:refnum<vi>, error out=w321:errorcluster)
            n180 = Index Array(array=w326, index=w325) -> (element=w324:enum16{"String", "Numeric"})
            n181 = Equal?(x=w311, y=w325) -> (x = y?=w329:bool)
            n182 = case shown="False" w329 {
              tunnel: w312 -> [w342 w352]
              tunnel: [FALSE ("Sorted AZ?") w351] -> w306
              tunnel: w321 -> [w346 w356]
              tunnel: [w345 w356] -> w328
              tunnel: w325 -> [w344 w355]
              tunnel: [w344 w355] -> w327
              tunnel: w311 -> [w343 _]
              tunnel: [w342 w354] -> w315
              tunnel: w311 -> [w341 _]
              tunnel: [w341 w353] -> w314
              tunnel: w310 -> [_ w354]
              tunnel: w309 -> [_ w353]
              frame False {
                # "New col, update secondaries"
                # "Make new sort column header bold\nand previous sort column header NOT bold"
                # "New col clicked, sort Ascending"
                n183 = property on="Data Tree" class="Tree (strict)"(error in=w346, "Active Item Tag"="TREE_COLUMN_HEADERS" ("Active Item:Tag"), "ActiveColNum"=w343, "CellFontBold"=FALSE ("Active Cell:Cell Font:Bold"), "ActiveColNum"=w344, "CellFontBold"=TRUE ("Active Cell:Cell Font:Bold")) -> (error out=w345:errorcluster)  [unwired: 1 in, 1 out]
              }
              frame True {
                # "Same col, maintain secondaries"
                # "Same col clicked, reverse order"
                n184 = Not(x=w352) -> (.not. x?=w351:bool)
              }
            }
            n185 = case shown="\"String\", Default" w324 {
              tunnel: [w335 w339] -> w318
              tunnel: w306 -> [w334 w338]
              tunnel: w328 -> [w333 w340]
              tunnel: w327 -> [w332 w336]
              tunnel: w313 -> [_ w337]
              frame "String", Default {
                n186 = invoke on="Data Tree" class="Tree (strict)" method="Edit Tree Items.Sort Children"(error in=w333, "Sort Column"=w332, "Sort Recursively"=TRUE ("Sort Recursively?"), "Reverse Order"=w334) -> (error out=w335:errorcluster)  [unwired: 4 in, 7 out]
              }
              frame "Numeric" {
                # "This col contains numeric\ndata and needs to be\nsorted suing special tricks\nas Tree:Sort method only\nsupports Alphabetical sorting."
                n187 = call "Sort Tree Items by Numerical order.vi"("Reverse Order?"=w338, "error in"=w340, "Sort Column"=w336, "Data Tree"=w337) -> ("error out"=w339:errorcluster)  [unwired: 7 in]
              }
            }
            n188 = Bundle By Name(cluster=w330, "SortOptions.RevDir.pri"=w306, "SortOptions.Col.pri"=w327, "SortOptions.RevDir.sec"=w315, "SortOptions.Col.sec"=w314) -> (w308:T2)
            n189 = property class="Pnl"(reference=w316, error in=w318, "DeferPanUpdts"=FALSE ("Defer Panel Updates")) -> (error out=w317:errorcluster)  [unwired: 1 out]
            n190 = call "Send Updated UI State to Processing Loop.vi"("Queue in"=w307, "ConfigInfo in"=w308) -> ()  [unwired: 9 in, 1 out]
          }
        }
      }
      event "Data Tree": Double Click {
        n191 = event-data() -> ("Tag"=w365:string)  [unwired: 1 out]
        n192 = Unbundle By Name(w357) -> ("Shared"=w359:refnum<data-value>)
        n193 = in-place {
          in-place-border: [w366] -> w358
          n194 = in-place-dvr #11(w359) -> (w367:T5)  [unwired: 1 out]
          n195 = Unbundle By Name(w367) -> ("App"=w366:refnum<vi>)
          n196 = in-place-dvr #11(w367) -> ()  [unwired: 2 out]
        }
        n197 = Open VI Reference(application reference (local)=w358, vi path=w365, error in (no error)=w364) -> (vi reference=w361:refnum<vi>, error out=w360:errorcluster)  [unwired: 3 out]
        n198 = Not A Number/Path/Refnum?(number/path/refnum=w361) -> (NaN/Path/Refnum?=w363:bool)
        n199 = case shown="False" w363 {
          tunnel: [w371 w394] -> w362
          tunnel: w361 -> [w370 _]
          tunnel: w360 -> [w369 w395]
          frame False {
            n200 = property class="VI"(reference=w370, error in=w369) -> (reference out=w372:refnum<vi>, error out=w373:errorcluster, "BDWin.Open"=w375:bool, "FP.State"=w374:T9)
            n201 = case shown="False" w375 {
              selector: w375 -> [_ w391]
              tunnel: w373 -> [w379 w392]
              tunnel: w374 -> [w380 _]
              tunnel: w372 -> [w378 w390]
              tunnel: [w377 w389] -> w368
              tunnel: [w376 w388] -> w371
              frame False {
                n202 = case shown="\"Standard\", Default" w380 {
                  tunnel: w379 -> [w381 w387]
                  tunnel: w378 -> [w382 w386]
                  tunnel: [w382 w385] -> w377
                  tunnel: [w381 w384] -> w376
                  frame "Invalid" {
                  }
                  frame "Standard", Default {
                    n203 = invoke class="VI" method="FP.Open"(reference=w386, error in=w387, "Activate"=TRUE ("Activate?")) -> (reference out=w385:refnum<vi>, error out=w384:errorcluster)  [unwired: 2 in, 3 out]
                  }
                }
              }
              frame True {
                # "Bring BD window to front"
                n204 = property class="VI"(reference=w390, error in=w392, "BDWin.Open"=w391) -> (reference out=w389:refnum<vi>, error out=w388:errorcluster)
              }
            }
            n205 = Close Reference(reference=w368) -> ()  [unwired: 1 in, 1 out]
          }
          frame True {
            # "Ignore errors when caused by double-click: \n* On a library item in tree (parents of VIs) [error 1004]\n* On Column Headers or empty tree area [error 1]"
            n206 = call-poly <vilib>:"Error_FilterCodes.vi"("error in (no error)"=w395, "Codes to filter"=i32[] [1, 1004]) -> ("error out"=w394:errorcluster)  [unwired: 9 in]
          }
        }
      }
      event User Event {
        # "If this is a Clone, mark it as the source of the pause event"
        n207 = event-data() -> ("VI"=w403:string)  [unwired: 1 out]
        n208 = Unbundle By Name(w397) -> ("Shared"=w398:refnum<data-value>)
        n209 = in-place {
          in-place-border: [w410] -> w396
          n210 = in-place-dvr #12(w398) -> (w411:T5)  [unwired: 1 out]
          n211 = Unbundle By Name(w411) -> ("App"=w410:refnum<vi>)
          n212 = in-place-dvr #12(w411) -> ()  [unwired: 2 out]
        }
        n213 = Open VI Reference(application reference (local)=w396, vi path=w403, error in (no error)=w402) -> (vi reference=w409:refnum<vi>, error out=w408:errorcluster)  [unwired: 3 out]
        n214 = property class="VI"(reference=w409, error in=w408) -> (reference out=w406:refnum<vi>, error out=w407:errorcluster, "IsCloneVI"=w404:bool)
        n215 = Close Reference(reference=w406, error in (no error)=w407) -> (error out=w405:errorcluster)
        n216 = case shown="True" w404 {
          tunnel: w403 -> [w419 w427]
          tunnel: [w420 w421] -> w400
          tunnel: w405 -> [_ _]
          frame False {
            n217 = Build Array(w419) -> (w420:string[])
          }
          frame True {
            # "VI that generated the Pause is a clone. Select all clones of the original VI."
            n218 = property on="Data Tree" class="Tree (strict)"() -> ("All Tags"=w422:string[])  [unwired: 2 in, 2 out]
            n219 = Search/Split String(string=w427, search string/char (-)=":") -> (substring before match=w423:string)  [unwired: 1 in, 2 out]
            n220 = for {
              shift-right: [w436] -> w425
              shift-left: w422 -> [w437]
              tunnel: w422 -> [w432] mode=indexing
              shift-right: [w435] -> w424
              shift-left: 0 -> [w434]
              tunnel: w423 -> [w429]
              n221 = Search/Split String(string=w432, search string/char (-)=":") -> (substring before match=w430:string, offset of match=w431:i32)  [unwired: 1 in, 1 out]
              n222 = case shown="0, Default" w431 {
                tunnel: w437 -> [w445 w454]
                tunnel: [w444 w454] -> w436
                tunnel: [w443 w453] -> w435
                tunnel: w434 -> [w442 w453]
                tunnel: w432 -> [w441 _]
                tunnel: w430 -> [w440 _]
                tunnel: w429 -> [w439 _]
                frame 0, Default {
                  n223 = Equal?(x=w439, y=w440) -> (x = y?=w438:bool)
                  n224 = case shown="True" w438 {
                    tunnel: w445 -> [w450 w452]
                    tunnel: [w447 w452] -> w444
                    tunnel: [w448 w451] -> w443
                    tunnel: w442 -> [w449 w451]
                    tunnel: w441 -> [w446 _]
                    frame True {
                      n225 = Increment(x=w449) -> (x+1=w448:i32)
                      n226 = Replace Array Subset(array=w450, new element=w446, index=w449) -> (w447:string[])
                    }
                    frame False {
                    }
                  }
                }
                frame -1 {
                }
              }
            }
            n227 = Array Subset(array=w425, length=w424) -> (w421:string[])  [unwired: 1 in]
          }
        }
        n228 = flat-sequence {
          tunnel: w400 -> [w412]
          tunnel: [w413] -> w399
          frame #0 {
            # "enforce"
            n229 = local write "Data Tree"(w412) -> ()
          }
          frame #1 {
            # "Call Pause event case to pause selected VIs"
            # "execution order"
            n230 = property on="Pause" class="Bool (strict)"("Val(Sgnl)"=TRUE ("Value (Signaling)")) -> (error out=w413:errorcluster)  [unwired: 2 in, 1 out]
          }
        }
        n231 = case shown="True" w404 {
          tunnel: w399 -> [w415 w418]
          tunnel: w403 -> [_ w417]
          tunnel: [w415 w416] -> w401
          frame False {
          }
          frame True {
            n232 = property on="Pause Source" class="Str"(error in=w418, "Val(Sgnl)"=w417) -> (error out=w416:errorcluster)  [unwired: 1 in, 1 out]
          }
        }
      }
      event User Event {
        n233 = event-data() -> ("source"=w461:string)  [unwired: 1 out]
        n234 = Concatenate Strings("!! Error in Task Manager !!\n\n" ("string"), w461) -> (w459:string)
        n235 = Two Button Dialog(message=w459, 1:"Ignore Error" ("F button name (\"Cancel\")"), 2:"End Task Manager" ("T button name (\"OK\")")) -> (T button?=w458:bool)
        n236 = case shown="True" w458 {
          selector: w458 -> [w465 w468]
          tunnel: [w465 w468] -> w457
          tunnel: w455 -> [_ w466]
          frame False {
          }
          frame True {
            n237 = Enqueue Element(queue=w466, element=cluster{"Command":string, "Data":variant} {"Command"="Exit", "Data"=variant}) -> ()  [unwired: 2 in, 3 out]
          }
        }
      }
      event Panel Close? {
        n238 = event-data() -> ()  [unwired: 2 out]
        n239 = call "Shutdown Progress Indicator.vi"() -> ()  [unwired: 11 in, 1 out]
        n240 = Enqueue Element(queue=w471, element=cluster{"Command":string, "Data":variant} {"Command"="Exit", "Data"=variant}, error in (no error)=w472) -> (error out=w469:errorcluster)  [unwired: 1 in, 2 out]
        n241 = event-data("Discard?"=TRUE) -> ()  [unwired: 1 in, 1 out]
      }
      event Key Down {
        # "#Verify Enable that pressing Ctrl+. will still Stop this top-level VI.  This is needed for during development."
        # "Enable Ctrl+. to stop this VI\nAllows to debug LVTM, by providing a mechanism to stop without exiting (useful during development)."
        n242 = event-data() -> ("ScanCode"=w477:i16, "PlatMods.Ctrl"=w476:bool)  [unwired: 9 out]
        n243 = Equal?(x=i16 52, y=w477) -> (x = y?=w479:bool)
        n244 = And(x=w479, y=w476) -> (x .and. y?=w478:bool)
        n245 = Stop(stop? (T)=w478) -> ()
      }
      event Menu Activation? {
        n246 = event-data() -> ("MenuRef"=w495:refnum<k9>)  [unwired: 1 out]
        n247 = Unbundle By Name(w483) -> ("Refresh Rate (ms)"=w482:i32)
        n248 = for {
          tunnel: string[] ["Paused", "High", "Normal", "Low"] -> [w511] mode=indexing
          tunnel: w482 -> [w510]
          tunnel: i32[] [-1, 200, 1000, 5000] -> [w508] mode=indexing
          tunnel: w492 -> [w507]
          tunnel: [w506] -> w491
          shift-right: [w505] -> w490
          shift-left: w495 -> [w512]
          n249 = Equal?(x=w508, y=w510) -> (x = y?=w509:bool)
          n250 = Set Menu Item Info(6:w509, 7:w511, 8:w507, 11:w512) -> (0:w506:errorcluster, 3:w505:refnum<k9>)  [unwired: 3 in]
        }
        n251 = Unbundle By Name(w483) -> ("View"=w489:T1)
        n252 = call "Update Filters Menu.vi"("error in"=w491, "ConfigInfo in"=w483, "Menu in"=w490) -> ("error out"=w486:errorcluster, "Menu out"=w488:refnum<k9>)  [unwired: 7 in]
        n253 = case shown="\"Flat List\"" w489 {
          tunnel: ["ViewGroupByLibrary" ("item tag") "ViewGroupByFolder" ("item tag") "ViewFlatList" ("item tag")] -> w484
          frame "Group By Library" {
          }
          frame "Group By Folder" {
          }
          frame "Flat List" {
          }
        }
        n254 = for {
          tunnel: w488 -> [w501]
          tunnel: string[] ["ViewGroupByLibrary", "ViewGroupByFolder", "ViewFlatList"] -> [w498] mode=indexing
          shift-right: [w500] -> w487
          shift-left: w486 -> [w499]
          tunnel: w484 -> [w497]
          n255 = Equal?(x=w498, y=w497) -> (x = y?=w496:bool)
          n256 = Set Menu Item Info(6:w496, 7:w498, 8:w499, 11:w501) -> (0:w500:errorcluster)  [unwired: 3 in, 1 out]
        }
        n257 = event-data() -> ()  [unwired: 2 in, 1 out]
      }
      event Menu Selection (User) {
        n258 = event-data() -> ("ItemTag"=w520:string, "MenuRef"=w518:refnum<k9>)  [unwired: 1 out]
        n259 = case shown="\"High\", \"Low\", \"Normal\", \"Paused\"" w520 {
          selector: w520 -> [_ _ w535 w543 w572 _ _ _ _ w662 _ w693 w704]
          tunnel: [_ TRUE ("stop") _ _ _ _ _ _ _ _ _ _ _] -> w519
          tunnel: w518 -> [_ _ _ w542 w571 _ _ _ _ _ _ _ _]
          tunnel: w515 -> [w522 w527 w534 w541 w570 w599 w602 w621 w642 w668 w679 w692 w708]
          tunnel: w517 -> [w521 w524 w530 w540 w569 w598 w601 w620 w641 w667 w682 w691 w707]
          tunnel: [w521 w523 w531 w540 w569 w598 w601 w620 w641 w658 w676 w683 w706] -> w516
          tunnel: [w522 w527 w532 w541 w570 w599 w602 w621 w642 w659 w677 w685 w702] -> w514
          tunnel: w513 -> [_ w525 w529 _ _ _ _ _ _ w665 w680 w686 w701]
          frame Default {
          }
          frame "Exit" {
            n260 = call "Shutdown Progress Indicator.vi"() -> ()  [unwired: 11 in, 1 out]
            n261 = Enqueue Element(queue=w525, element=cluster{"Command":string, "Data":variant} {"Command"="Exit", "Data"=variant}, error in (no error)=w524) -> (error out=w523:errorcluster)  [unwired: 1 in, 2 out]
          }
          frame "High", "Low", "Normal", "Paused" {
            n262 = case shown="\"Normal\", Default" w535 {
              tunnel: [5000 ("Value (Signaling)") 1000 ("Value (Signaling)") 200 ("Value (Signaling)") -1 ("Value (Signaling)")] -> w533
              frame "Low" {
              }
              frame "Normal", Default {
              }
              frame "High" {
              }
              frame "Paused" {
              }
            }
            n263 = Bundle By Name(cluster=w534, "Refresh Rate (ms)"=w533) -> (w532:T2)
            n264 = call "Send Updated UI State to Processing Loop.vi"("error in (no error)"=w530, "Queue in"=w529, "ConfigInfo in"=w532) -> ("error out"=w531:errorcluster)  [unwired: 8 in]
          }
          frame "Find" {
            n265 = disable-structure shown="ENABLE_FIND_FILTER==False, Default" {
              disable-tunnel: w543 -> [_ w552]
              disable-tunnel: w542 -> [_ w549]
              frame condition #0 (active) {
                w545 = 1000  # timeout (ms)
                # "#ToDo These features are a work in progress, and are not yet ready for prime-time.\n-- TimVargo"
                n266 = call "MsgBalloon.vi"("timeout (ms)"=w545, "strCaption"="Find Item Name", "strText"="function is not yet implimented") -> ()  [unwired: 8 in, 1 out]
              }
              frame condition #1 {
                # "update checkmarks"
                n267 = local read "FindIsActive"() -> (w551:bool)
                n268 = Not(x=w551) -> (.not. x?=w553:bool)
                n269 = Set Menu Item Info(6:FALSE ("checked"), 7:"FilterOnName" ("item tag"), 11:w549) -> ()  [unwired: 4 in, 2 out]
                n270 = Set Menu Item Info(6:w553, 7:w552, 11:w549) -> ()  [unwired: 4 in, 2 out]
                n271 = case shown="False" w551 {
                  selector: w551 -> [w562 w568]
                  tunnel: [w561 w565] -> w554
                  tunnel: [w560 w567] -> _
                  tunnel: [w556 w565] -> w550
                  frame False {
                    w559 = path "Dynamic_FindName_LVTM/FindNameInTree.vi"  # function path
                    # "3. invoke find"
                    # "1. stop the Filter function"
                    # "start the Find tool"
                    # "2. toggle the Find status"
                    n272 = control-ref of="ToolPanel"() -> (w558:refnum<vi>)
                    n273 = control-ref of="Data Tree"() -> (w563:refnum<vi>)
                    n274 = call "StopLooking.vi"("stop notif name"="StopFilterNotification", "SubPanel in"=w558) -> ("StopAck"=w556:bool, "SubPanel out"=w557:refnum<vi>)  [unwired: 7 in, 1 out]
                    n275 = Not(x=w562) -> (.not. x?=w561:bool)
                    n276 = call "Dispatch_FindOrFilterOnName.vi"("function path"=w559, "Data Tree in"=w563, "SubPanel in"=w557) -> ("error out"=w560:errorcluster)  [unwired: 6 in, 2 out]
                  }
                  frame True {
                    # "1. stop the Find function & remove the Find UI"
                    # "stop the Find tool"
                    # "2. toggle the Find status, force the Filter status false"
                    n277 = control-ref of="ToolPanel"() -> (w566:refnum<vi>)
                    n278 = call "StopLooking.vi"("stop notif name"="StopFindNotification", "SubPanel in"=w566) -> ("error out"=w567:errorcluster)  [unwired: 7 in, 2 out]
                    n279 = Not(x=w568) -> (.not. x?=w565:bool)
                  }
                }
                n280 = local write "FindIsActive"(w554) -> ()
                n281 = local write "NameFilterIsActive"(w550) -> ()
              }
            }
          }
          frame "FilterOnName" {
            n282 = disable-structure shown="ENABLE_FIND_FILTER==TRUE" {
              disable-tunnel: w572 -> [_ w582]
              disable-tunnel: w571 -> [_ w577]
              frame condition #0 (active) {
                w573 = 1000  # timeout (ms)
                # "#ToDo These features are a work in progress, and are not yet ready for prime-time.\n-- TimVargo"
                n283 = call "MsgBalloon.vi"("timeout (ms)"=w573, "strCaption"="Filter On Name", "strText"="function is not yet implimented") -> ()  [unwired: 8 in, 1 out]
              }
              frame condition #1 {
                # "update checkmarks"
                n284 = local read "NameFilterIsActive"() -> (w581:bool)
                n285 = Not(x=w581) -> (.not. x?=w583:bool)
                n286 = Set Menu Item Info(6:FALSE ("checked"), 7:"Find" ("item tag"), 11:w577) -> ()  [unwired: 4 in, 2 out]
                n287 = Set Menu Item Info(6:w583, 7:w582, 11:w577) -> ()  [unwired: 4 in, 2 out]
                n288 = case shown="False" w581 {
                  selector: w581 -> [w592 w597]
                  tunnel: [w589 w596] -> _
                  tunnel: [w591 w594] -> w580
                  tunnel: [w584 w594] -> w579
                  frame False {
                    w588 = path "Dynamic_FindName_LVTM/FilterOnNameInTree.vi"  # function path
                    # "3. invoke filter"
                    # "1. stop the Find function"
                    # "start the FilterOnName tool"
                    # "2. toggle the Filter status"
                    n289 = control-ref of="ToolPanel"() -> (w587:refnum<vi>)
                    n290 = control-ref of="Data Tree"() -> (w590:refnum<vi>)
                    n291 = call "StopLooking.vi"("stop notif name"="StopFindNotification", "SubPanel in"=w587) -> ("StopAck"=w584:bool, "SubPanel out"=w585:refnum<vi>)  [unwired: 7 in, 1 out]
                    n292 = Not(x=w592) -> (.not. x?=w591:bool)
                    n293 = call "Dispatch_FindOrFilterOnName.vi"("function path"=w588, "Data Tree in"=w590, "SubPanel in"=w585) -> ("error out"=w589:errorcluster)  [unwired: 6 in, 2 out]
                  }
                  frame True {
                    # "1. stop the FilterOnName function & remove the Filter UI"
                    # "stop the FilterOnName tool"
                    # "2. toggle the Filter status, force the Find status false"
                    n294 = control-ref of="ToolPanel"() -> (w595:refnum<vi>)
                    n295 = call "StopLooking.vi"("stop notif name"="StopFilterNotification", "SubPanel in"=w595) -> ("error out"=w596:errorcluster)  [unwired: 7 in, 2 out]
                    n296 = Not(x=w597) -> (.not. x?=w594:bool)
                  }
                }
                n297 = local write "NameFilterIsActive"(w580) -> ()
                n298 = local write "FindIsActive"(w579) -> ()
              }
            }
          }
          frame "Refresh Now" {
            n299 = property on="Refresh" class="Bool (strict)"("Val(Sgnl)"=TRUE ("Value (Signaling)")) -> ()  [unwired: 2 in, 2 out]
          }
          frame "UserTools" {
            n300 = disable-structure shown="ENABLE_FIND_FILTER==FALSE, Default" {
              disable-tunnel: w602 -> [w616 _]
              frame condition #0 {
                # "#ToDo This will likely need some additional logic, to make it work in the toolkit environment.  In any case, the intent is to eventually use a plug-in architecture here."
                # "Prepare to call and forget"
                n301 = Current VI's Path() -> (path=w606:path)
                n302 = Strip Path(path=w606) -> (stripped path=w603:path)  [unwired: 1 out]
                n303 = Unbundle By Name(w616) -> ("AppInst"=w607)
                n304 = Build Path(base path=w603, name or relative path=path "Utils_LVTM/DiscoverCommonTypeDefCallers.vi" ("vi path")) -> (appended path=w604:path)
                n305 = vi-ref "DiscoverCommonTypeDefCallers.vi"() -> (w615:refnum<vi>)
                n306 = Open VI Reference(type specifier VI Refnum (for type only)=w615, application reference (local)=w607, vi path=w604, options=128) -> (vi reference=w611:refnum<vi>, error out=w612:errorcluster)  [unwired: 2 in]
                n307 = call-by-ref "Start Asynchronous Call"(reference=w611, error in=w612, "Application Reference"=w607) -> (reference out=w610:refnum<vi>, error out=w609:errorcluster)  [unwired: 9 in, 2 out]
                n308 = invoke class="VI (strict)" method="FP.Open"(reference=w610, error in=w609) -> (reference out=w614:refnum<vi>, error out=w613:errorcluster)  [unwired: 3 in, 3 out]
                n309 = Close Reference(reference=w614, error in (no error)=w613) -> ()  [unwired: 1 out]
              }
              frame condition #1 (active) {
                w617 = 1000  # timeout (ms)
                # "#ToDo These features are a work in progress, and are not yet ready for prime-time.\n-- TimVargo"
                n310 = call "MsgBalloon.vi"("timeout (ms)"=w617, "strCaption"="User Tools", "strText"="function is not yet implimented") -> ()  [unwired: 8 in, 1 out]
              }
            }
          }
          frame "HelpAboutInfo" {
            # "#Verify Fixed, path is not correct when deployed"
            # "Detect if this tool is running as a deployed toolkit.  Most toolkits, including this one, are located on disk below the 'project' directory of each LV version.  This is also NI's recommended 'best practice'."
            n311 = VI Library() -> (path=w623:path)
            n312 = Build Path(base path=w623, name or relative path="..\\project\\") -> (appended path=w631:path)
            n313 = Current VI's Path() -> (path=w629:path)
            n314 = Path to Array of Strings(0:w629) -> (2:w626:string[])  [unwired: 1 out]
            n315 = Path to Array of Strings(0:w631) -> (2:w628:string[])  [unwired: 1 out]
            n316 = Array Size(array=w628) -> (size(s)=w627:i32)
            n317 = Array Subset(array=w626, length=w627) -> (w625:string[])  [unwired: 1 in]
            n318 = Array of Strings to Path(0:w625) -> (2:w624:path)  [unwired: 1 in]
            n319 = Equal?(x=w624, y=w631) -> (x = y?=w622:bool)
            n320 = case shown="True" w622 {
              tunnel: [w633 w635] -> w632
              frame True {
                # "LV Toolkit path"
                n321 = call <userlib>:"VI Library__ogtk.vi"("Relative path (.)"=path "LAVA/LVTM/Documentation" ("name or relative path")) -> ("VI Library (+ Relative)"=w633:path)
              }
              frame False {
                # "Development path"
                n322 = call <userlib>:"Current VIs Parent Directory__ogtk.vi"("Relative path (.)"=path "Documentation" ("name or relative path")) -> ("Parent Directory (+ Relative)"=w635:path)  [unwired: 4 in]
              }
            }
            n323 = call "RHA_dialog.vi"("DocFolder"=w632) -> ()  [unwired: 11 in]
          }
          frame "UserGuide" {
            # "Detect if this tool is running as a deployed toolkit.  Most toolkits, including this one, are located on disk below the 'project' directory of each LV version.  This is also NI's recommended 'best practice'."
            n324 = VI Library() -> (path=w644:path)
            n325 = Build Path(base path=w644, name or relative path="..\\project\\") -> (appended path=w652:path)
            n326 = Current VI's Path() -> (path=w650:path)
            n327 = Path to Array of Strings(0:w650) -> (2:w647:string[])  [unwired: 1 out]
            n328 = Path to Array of Strings(0:w652) -> (2:w649:string[])  [unwired: 1 out]
            n329 = Array Size(array=w649) -> (size(s)=w648:i32)
            n330 = Array Subset(array=w647, length=w648) -> (w646:string[])  [unwired: 1 in]
            n331 = Array of Strings to Path(0:w646) -> (2:w645:path)  [unwired: 1 in]
            n332 = Equal?(x=w645, y=w652) -> (x = y?=w643:bool)
            n333 = case shown="True" w643 {
              tunnel: [w653 w655] -> w639
              frame True {
                # "LV Toolkit path"
                n334 = call <userlib>:"VI Library__ogtk.vi"("Relative path (.)"=path "LAVA/LVTM/Documentation" ("name or relative path")) -> ("VI Library (+ Relative)"=w653:path)
              }
              frame False {
                # "Development path"
                n335 = call <userlib>:"Current VIs Parent Directory__ogtk.vi"("Relative path (.)"=path "Documentation" ("name or relative path")) -> ("Parent Directory (+ Relative)"=w655:path)  [unwired: 4 in]
              }
            }
            n336 = Build Path(base path=w639, name or relative path="Manual.pdf") -> (appended path=w637:path)
            n337 = call <vilib>:"Open a Document on Disk.vi"("document path"=w637) -> ("error out"=w640:errorcluster)  [unwired: 6 in]
            n338 = call <vilib>:"Simple Error Handler.vi"("error in (no error)"=w640) -> ()  [unwired: 4 in, 5 out]
          }
          frame "FilterExtension_A".."FilterExtension_z" {
            n339 = Unbundle By Name(w668) -> ("File Extension Filters"=w664:string[])
            n340 = Match Pattern(string=w662, regular expression="FilterExtension_") -> (after substring=w660:string)  [unwired: 1 in, 3 out]
            n341 = Search 1D Array(1D array=w664, element=w660) -> (index of element=w663:i32)  [unwired: 1 in]
            n342 = case shown="-1" w663 {
              selector: w663 -> [w669 _]
              tunnel: w664 -> [w671 w674]
              tunnel: w660 -> [_ w673]
              tunnel: [w670 w672] -> w666
              frame 0, Default {
                # "Filter for this extension exists.\nRemove it"
                n343 = Delete From Array(array=w671, index=w669) -> (array with subset deleted=w670:string[])  [unwired: 1 in, 1 out]
              }
              frame -1 {
                # "Filter for this extension doesn't exist.\nAdd it."
                n344 = Build Array (concatenate)(w674, w673) -> (w672:string[])
              }
            }
            n345 = Bundle By Name(cluster=w668, "File Extension Filters"=w666) -> (w659:T2)
            n346 = call "Request Processing Loop to Refresh Tree.vi"("error in (no error)"=w667, "Queue in"=w665, "ConfigInfo in"=w659) -> ("error out"=w657:errorcluster)  [unwired: 8 in]
            n347 = call "Update Active Filters.vi"("error in"=w657, "Configuration"=w659) -> ("error out"=w658:errorcluster)  [unwired: 9 in]
          }
          frame "FilterType_Global" {
            n348 = Unbundle By Name(w679) -> ("Filter Global VIs"=w678:bool)
            n349 = Not(x=w678) -> (.not. x?=w681:bool)
            n350 = Bundle By Name(cluster=w679, "Filter Global VIs"=w681) -> (w677:T2)
            n351 = call "Request Processing Loop to Refresh Tree.vi"("error in (no error)"=w682, "Queue in"=w680, "ConfigInfo in"=w677) -> ("error out"=w675:errorcluster)  [unwired: 8 in]
            n352 = call "Update Active Filters.vi"("error in"=w675, "Configuration"=w677) -> ("error out"=w676:errorcluster)  [unwired: 9 in]
          }
          frame "FilterPath_A".."FilterPath_z" {
            n353 = Match Pattern(string=w693, regular expression="FilterPath_" ("menu tag")) -> (after substring=w687:string)  [unwired: 1 in, 3 out]
            n354 = case shown="Default" w687 {
              selector: w687 -> [_ w695]
              tunnel: w692 -> [w694 w696]
              tunnel: [_ w699] -> w690
              tunnel: [w694 w696] -> w688
              frame "RemoveAll" {
              }
              frame Default {
                n355 = Unbundle By Name(w696) -> ("Filtered Paths"=w700:path[])
                n356 = String To Path(string=w695) -> (path=w697:path)
                n357 = Search 1D Array(1D array=w700, element=w697) -> (index of element=w698:i32)  [unwired: 1 in]
                n358 = Delete From Array(array=w700, index=w698) -> (array with subset deleted=w699:path[])  [unwired: 1 in, 1 out]
              }
            }
            n359 = Bundle By Name(cluster=w688, "Filtered Paths"=w690) -> (w685:T2)
            n360 = call "Request Processing Loop to Refresh Tree.vi"("error in (no error)"=w691, "Queue in"=w686, "ConfigInfo in"=w685) -> ("error out"=w684:errorcluster)  [unwired: 8 in]
            n361 = call "Update Active Filters.vi"("error in"=w684, "Configuration"=w685) -> ("error out"=w683:errorcluster)  [unwired: 9 in]
          }
          frame "ViewFlatList", "ViewGroupByFolder", "ViewGroupByLibrary" {
            n362 = case shown="\"ViewGroupByLibrary\"" w704 {
              tunnel: w708 -> [w710 w712 w714]
              tunnel: [View."Flat List" ("View") View."Group By Library" ("View") View."Group By Folder" ("View")] -> w703
              tunnel: [w710 w712 w714] -> w705
              frame "ViewFlatList", Default {
              }
              frame "ViewGroupByLibrary" {
              }
              frame "ViewGroupByFolder" {
              }
            }
            n363 = Bundle By Name(cluster=w705, "View"=w703) -> (w702:T2)
            n364 = local write "View"(w703) -> ()
            n365 = call "Request Processing Loop to Refresh Tree.vi"("error in (no error)"=w707, "Queue in"=w701, "ConfigInfo in"=w702) -> ("error out"=w706:errorcluster)  [unwired: 8 in]
          }
        }
      }
      event "Data Tree": Shortcut Menu Activation? {
        n366 = event-data() -> ("MenuRef"=w724:refnum<k9>, "CtlRef"=w723:refnum<vi>, "Coords"=w722:T8)  [unwired: 1 out]
        n367 = invoke class="Tree (strict)" method="Point To Row Column"(reference=w723, error in=w719, "Point"=w722) -> (reference out=w721:refnum<vi>, error out=w720:errorcluster, "Tag"=w716:string)  [unwired: 5 in, 5 out]
        n368 = case shown="Default" w716 {
          selector: w716 -> [w725 _]
          tunnel: w724 -> [w732 _]
          tunnel: w721 -> [w731 _]
          tunnel: w720 -> [w730 _]
          tunnel: w718 -> [w728 _]
          tunnel: [w726 _] -> w717
          tunnel: [_ TRUE ("Discard?")] -> w715
          frame Default {
            n369 = property class="Tree (strict)"(reference=w731, error in=w730, "Active Item Tag"=w725) -> (error out=w727:errorcluster, "Child-Only?"=w729:bool)  [unwired: 1 out]
            n370 = case shown="False" w729 {
              tunnel: w732 -> [w737 _]
              tunnel: w728 -> [w736 _]
              tunnel: w727 -> [w734 w744]
              tunnel: [w733 w744] -> w726
              frame False {
                n371 = Unbundle By Name(w736) -> ("View"=w735:T1)
                n372 = case shown="\"Group By Folder\"" w735 {
                  tunnel: w737 -> [_ w743]
                  tunnel: w734 -> [w738 w740]
                  tunnel: [w738 w739] -> w733
                  frame "Group By Library", Default {
                  }
                  frame "Group By Folder" {
                    n373 = Insert Menu Items(6:w740, 7:string[] ["APP_SEPARATOR", "ExcludeThisFolder", "ExcludeAllButThisFolder"] ("item tags"), 8:string[] ["APP_SEPARATOR", "Filter Out This Folder", "Filter Out All But This Folder"] ("item names"), 9:w743) -> (0:w739:errorcluster)  [unwired: 2 in, 2 out]
                  }
                }
              }
              frame True {
              }
            }
          }
          frame "", "TREE_COLUMN_HEADERS" {
          }
        }
        n374 = event-data("Discard?"=w715) -> ()  [unwired: 1 in, 1 out]
      }
      event "Data Tree": Shortcut Menu Selection (User) {
        n375 = event-data() -> ("CtlRef"=w746:refnum<vi>, "ItemTag"=w748:string, "Coords"=w747:T8)  [unwired: 1 out]
        n376 = case shown="\"ExcludeAllButThisFolder\", \"ExcludeThisFolder\"" w748 {
          selector: w748 -> [w757 w795]
          tunnel: w752 -> [w771 w802]
          tunnel: w751 -> [w768 w796]
          tunnel: [w754 w800] -> w750
          tunnel: [w760 w796] -> w749
          tunnel: w747 -> [w770 _]
          tunnel: w746 -> [w769 _]
          frame "ExcludeAllButThisFolder", "ExcludeThisFolder" {
            # "Keep only those items from tracking that still exist in the tree after deleting this folder."
            n377 = invoke class="Tree (strict)" method="Point To Row Column"(reference=w769, error in=w771, "Point"=w770) -> (reference out=w765:refnum<vi>, error out=w763:errorcluster, "Tag"=w764:string)  [unwired: 5 in, 5 out]
            n378 = case shown="\"ExcludeAllButThisFolder\"" w757 {
              tunnel: w765 -> [w783 w793]
              tunnel: w764 -> [w784 w792]
              tunnel: w763 -> [w786 w791]
              tunnel: [w781 w789] -> w762
              tunnel: [w785 w788] -> w761
              tunnel: [w782 w787] -> w758
              frame "ExcludeAllButThisFolder" {
                n379 = call "Delete All But Current Folder Hierarchy.vi"("error in"=w786, "Item Tag"=w784, "TreeControl in"=w783) -> ("error out"=w785:errorcluster, "Deleted Folders"=w782:path[], "TreeControl out"=w781:refnum<vi>)  [unwired: 6 in]
              }
              frame "ExcludeThisFolder", Default {
                # "Delete the item from the tree"
                n380 = String To Path(string=w792) -> (path=w794:path)
                n381 = invoke class="Tree (strict)" method="Edit Tree Items.Delete"(reference=w793, error in=w791, "tag"=w792, "Delete Children"=TRUE ("Delete Children?")) -> (reference out=w789:refnum<vi>, error out=w788:errorcluster)  [unwired: 1 in, 3 out]
                n382 = Build Array(w794) -> (w787:path[])
              }
            }
            n383 = Unbundle By Name(w768) -> ("Filtered Paths"=w767:path[], "Shared"=w756:refnum<data-value>)
            n384 = property class="Tree (strict)"(reference=w762, error in=w761) -> (error out=w759:errorcluster, "All Tags"=w755:string[])  [unwired: 1 out]
            n385 = Build Array (concatenate)(w767, w758) -> (w766:path[])
            n386 = Bundle By Name(cluster=w768, "Filtered Paths"=w766) -> (w760:T2)
            n387 = in-place {
              in-place-border: w755 -> [w772]
              n388 = in-place-dvr #13(w756) -> (w776:T5)  [unwired: 1 out]
              n389 = Unbundle By Name(w776) -> ("VIs"=w774:string[])
              n390 = for {
                tunnel: w774 -> [w780] mode=indexing
                tunnel: [w780] -> w773 mode=indexing if=w777
                tunnel: w772 -> [w779]
                n391 = Search 1D Array(1D array=w779, element=w780) -> (index of element=w778:i32)  [unwired: 1 in]
                n392 = Greater Or Equal To 0?(x=w778) -> (x >= 0?=w777:bool)
              }
              n393 = Bundle By Name(cluster=w776, "VIs"=w773) -> (w775:T5)
              n394 = in-place-dvr #13(w775) -> (w753:errorcluster)  [unwired: 1 out]
            }
            n395 = Merge Errors(w759, w753) -> (w754:errorcluster)
          }
          frame Default {
            n396 = case shown="\"AbortVI\"" w795 {
              selector: w795 -> [w814 _ _ _ _ _ _ _ _ _ _ _ _ _ w876]
              tunnel: w802 -> [_ w817 w820 w823 w826 w829 w832 w835 w838 w841 w844 w848 w851 w859 w879]
              tunnel: [_ w818 w821 w824 w827 w830 w833 w836 w839 w842 w845 w847 w850 w857 w877] -> w801
              tunnel: w796 -> [_ _ _ _ _ _ _ _ _ _ _ _ _ w853 w872]
              tunnel: [_ _ _ _ _ _ _ _ _ _ _ _ _ w856 w874] -> w798
              frame Default {
                w816 = 1000  # timeout (ms)
                # "do nothing"
                n397 = Format Into String(format string="Right-click %s" ("strCaption"), w814) -> (resulting string=w812:string)  [unwired: 2 in, 1 out]
                n398 = call "MsgBalloon.vi"("timeout (ms)"=w816, "strCaption"=w812, "strText"="function is not yet implimented") -> ()  [unwired: 8 in, 1 out]
              }
              frame "PauseExecution" {
                n399 = property on="Pause" class="Bool (strict)"(error in=w817, "Val(Sgnl)"=TRUE ("Value (Signaling)")) -> (error out=w818:errorcluster)  [unwired: 1 in, 1 out]
              }
              frame "ResumeExecution" {
                n400 = property on="Resume" class="Bool (strict)"(error in=w820, "Val(Sgnl)"=TRUE ("Value (Signaling)")) -> (error out=w821:errorcluster)  [unwired: 1 in, 1 out]
              }
              frame "TogglePauseExecution" {
                n401 = property on="Toggle Pause" class="Bool (strict)"(error in=w823, "Val(Sgnl)"=TRUE ("Value (Signaling)")) -> (error out=w824:errorcluster)  [unwired: 1 in, 1 out]
              }
              frame "HighlightExecution" {
                n402 = property on="Highlight Execution" class="Bool (strict)"(error in=w826, "Val(Sgnl)"=TRUE ("Value (Signaling)")) -> (error out=w827:errorcluster)  [unwired: 1 in, 1 out]
              }
              frame "DoNotHighlightExecution" {
                n403 = property on="Do Not Highlight Execution" class="Bool (strict)"(error in=w829, "Val(Sgnl)"=TRUE ("Value (Signaling)")) -> (error out=w830:errorcluster)  [unwired: 1 in, 1 out]
              }
              frame "AbortVI" {
                n404 = property on="Abort" class="Bool (strict)"(error in=w832, "Val(Sgnl)"=TRUE ("Value (Signaling)")) -> (error out=w833:errorcluster)  [unwired: 1 in, 1 out]
              }
              frame "OpenFP" {
                n405 = property on="Open Front Panel" class="Bool (strict)"(error in=w835, "Val(Sgnl)"=TRUE ("Value (Signaling)")) -> (error out=w836:errorcluster)  [unwired: 1 in, 1 out]
              }
              frame "CloseFP" {
                n406 = property on="Close Front Panel" class="Bool (strict)"(error in=w838, "Val(Sgnl)"=TRUE ("Value (Signaling)")) -> (error out=w839:errorcluster)  [unwired: 1 in, 1 out]
              }
              frame "OpenBD" {
                n407 = property on="Open Block Diagram" class="Bool (strict)"(error in=w841, "Val(Sgnl)"=TRUE ("Value (Signaling)")) -> (error out=w842:errorcluster)  [unwired: 1 in, 1 out]
              }
              frame "CloseBD" {
                n408 = property on="Close Block Diagram" class="Bool (strict)"(error in=w844, "Val(Sgnl)"=TRUE ("Value (Signaling)")) -> (error out=w845:errorcluster)  [unwired: 1 in, 1 out]
              }
              frame "TREE_OPEN_ALL_ITEMS" {
                n409 = invoke on="Data Tree" class="Tree (strict)" method="Open/Close.Open/Close All"(error in=w848, "Open"=TRUE ("Open?")) -> (error out=w847:errorcluster)  [unwired: 2 in, 3 out]
              }
              frame "TREE_CLOSE_ALL_ITEMS" {
                n410 = invoke on="Data Tree" class="Tree (strict)" method="Open/Close.Open/Close All"(error in=w851, "Open"=FALSE ("Open?")) -> (error out=w850:errorcluster)  [unwired: 2 in, 3 out]
              }
              frame "NonReentrant" {
                n411 = Unbundle By Name(w853) -> ("Shared"=w855:refnum<data-value>)
                n412 = in-place {
                  in-place-border: [w860] -> w854
                  n413 = in-place-dvr #14(w855) -> (w861:T5)  [unwired: 1 out]
                  n414 = Unbundle By Name(w861) -> ("App"=w860:refnum<vi>)
                  n415 = in-place-dvr #14(w861) -> ()  [unwired: 2 out]
                }
                n416 = local read "Data Tree"() -> (w856:string[])
                n417 = for {
                  tunnel: [w870] -> w858 mode=indexing
                  tunnel: w859 -> [w869]
                  tunnel: w856 -> [w868] mode=indexing
                  tunnel: w854 -> [w863]
                  n418 = Open VI Reference(application reference (local)=w863, vi path=w868, error in (no error)=w869) -> (vi reference=w866:refnum<vi>, error out=w867:errorcluster)  [unwired: 3 out]
                  n419 = property class="VI"(reference=w866, error in=w867, "Exec.IsReentrant"=FALSE ("Execution:Is Reentrant")) -> (reference out=w865:refnum<vi>, error out=w864:errorcluster)
                  n420 = Close Reference(reference=w865, error in (no error)=w864) -> (error out=w870:errorcluster)
                }
                n421 = Merge Errors(w858) -> (w857:errorcluster)
              }
              frame "PreallocatedClone", "SharedClone" {
                n422 = Unbundle By Name(w872) -> ("Shared"=w873:refnum<data-value>)
                n423 = case shown="\"PreallocatedClone\", Default" w876 {
                  tunnel: [T6."Preallocate clone for each instance" ("Execution:Reentrancy Type") T6."Share clones between instances" ("Execution:Reentrancy Type")] -> w875
                  frame "PreallocatedClone", Default {
                  }
                  frame "SharedClone" {
                  }
                }
                n424 = in-place {
                  in-place-border: [w880] -> w871
                  n425 = in-place-dvr #15(w873) -> (w881:T5)  [unwired: 1 out]
                  n426 = Unbundle By Name(w881) -> ("App"=w880:refnum<vi>)
                  n427 = in-place-dvr #15(w881) -> ()  [unwired: 2 out]
                }
                n428 = local read "Data Tree"() -> (w874:string[])
                n429 = for {
                  tunnel: [w893] -> w878 mode=indexing
                  tunnel: w879 -> [w892]
                  tunnel: w874 -> [w891] mode=indexing
                  tunnel: w871 -> [w886]
                  tunnel: w875 -> [w884]
                  n430 = Open VI Reference(application reference (local)=w886, vi path=w891, error in (no error)=w892) -> (vi reference=w889:refnum<vi>, error out=w890:errorcluster)  [unwired: 3 out]
                  n431 = property class="VI"(reference=w889, error in=w890, "Exec.IsReentrant"=TRUE ("Execution:Is Reentrant"), "Exec.ReentrancyType"=w884) -> (reference out=w888:refnum<vi>, error out=w887:errorcluster)
                  n432 = Close Reference(reference=w888, error in (no error)=w887) -> (error out=w893:errorcluster)
                }
                n433 = Merge Errors(w878) -> (w877:errorcluster)
              }
            }
            n434 = Empty Array?(array=w798) -> (empty?=w797:bool)
            n435 = case shown="False" w797 {
              tunnel: w798 -> [w809 _]
              tunnel: w796 -> [w805 _]
              tunnel: [w806 _] -> w799
              frame False {
                # "Update all properties for the selected items"
                n436 = Unbundle By Name(w805) -> ("Shared"=w803:refnum<data-value>, "Data Tree Ref"=w808:refnum<vi>)
                n437 = in-place {
                  in-place-border: [w810] -> w804
                  n438 = in-place-dvr #16(w803) -> (w811:T5)  [unwired: 1 out]
                  n439 = Unbundle By Name(w811) -> ("App"=w810:refnum<vi>)
                  n440 = in-place-dvr #16(w811) -> ()  [unwired: 2 out]
                }
                n441 = call "Update Tree Items.vi"("Properties"=enum16{"All", "Dynamic"}."All", "All Tags"=w809, "Data Tree Ref"=w808, "AppInst"=w804) -> ("error out"=w806:errorcluster)  [unwired: 7 in]
              }
              frame True {
              }
            }
            n442 = Merge Errors(w801, w799) -> (w800:errorcluster)
          }
        }
      }
    }
    n443 = call "Report Error.vi"("error in"=w30) -> ("error out"=w29:errorcluster)  [unwired: 10 in]
  }
  n444 = Enqueue Element(queue=w7, element=cluster{"Command":string, "Data":variant} {"Command"="Initialize", "Data"=variant}, error in (no error)=w5) -> (queue out=w6:refnum<queue>, error out=w4:errorcluster)  [unwired: 1 in, 1 out]
  n445 = while {
    tunnel: w4 -> [w903]
    shift-right: [w905] -> _
    shift-left: T3 {"Shared"=refnum, "Plugins"=[], "UIConfig"={"Data Tree Ref"=refnum, "FP Ref"=refnum, "Column Data Type"=[], "Search Clones Up To"=100, "SortOptions"={"Col.pri"=0, "RevDir.pri"=FALSE, "Col.sec"=0, "RevDir.sec"=FALSE}, "Group/Flat (0:group)"=FALSE, "CollapsedNodes"=[], "Show/Hide Cols"=[], "Filtered Paths"=[], "View"=enum."Group By Library", "File Extension Filters"=[], "Filter Global VIs"=FALSE, "Shared"=refnum, "Active Filters"=refnum, "Refresh Rate (ms)"=0}} -> [w895]
    tunnel: w6 -> [w904]
    tunnel: [w896] -> w2
    stop <- w898 stop-if-true
    # "Processing Loop"
    n446 = Unbundle By Name(w895) -> ("UIConfig.Refresh Rate (ms)"=w894:i32)
    n447 = Dequeue Element(queue=w904, timeout in ms (-1)=w894, error in (no error)=w903) -> (queue out=w897:refnum<queue>, element=w900:cluster{"Command":string, "Data":variant}, timed out?=w901:bool, error out=w902:errorcluster)
    n448 = case shown="False" w901 {
      tunnel: w895 -> [w911 w955]
      tunnel: w902 -> [w908 w953]
      tunnel: [w912 w955] -> w905
      tunnel: [w909 w952] -> w899
      tunnel: w900 -> [w914 _]
      tunnel: [w907 _] -> w898
      tunnel: w897 -> [w906 _]
      frame False {
        # "Received a command"
        n449 = Unbundle(w914) -> ("Command"=w913:string, "Data"=w910:variant)
        n450 = case shown="\"Refresh View\"" w913 {
          tunnel: [w916 w921 w925 w938 w944] -> w912
          tunnel: w911 -> [w916 w923 w933 w935 w944]
          tunnel: w910 -> [_ _ w932 w940 _]
          tunnel: [w915 w919 w927 w937 w946] -> w909
          tunnel: w908 -> [w915 w920 w931 w939 w945]
          tunnel: [_ _ _ _ TRUE] -> w907
          tunnel: w906 -> [_ _ _ _ w947]
          frame "", Default {
          }
          frame "Initialize" {
            n451 = call-dynamic "Launch.vi"("error in (no error)"=w920, "TCP_Server in"=refnum<class "TCP_Server.lvclass"> refnum) -> ("error out"=w919:errorcluster, "TCP_Server out"=w918:refnum<class "TCP_Server.lvclass">)  [unwired: 8 in]
            n452 = Build Array(w918) -> (w917:refnum<class "TCP_Server.lvclass">[])
            n453 = Bundle By Name(cluster=w923, "Plugins"=w917) -> (w921:T3)
          }
          frame "Refresh View" {
            n454 = Variant To Data(error in=w931, type=cluster{"UI State":T2, "Force Update":bool} {"UI State"={"Data Tree Ref"=refnum, "FP Ref"=refnum, "Column Data Type"=[], "Search Clones Up To"=0, "SortOptions"={"Col.pri"=0, "RevDir.pri"=FALSE, "Col.sec"=0, "RevDir.sec"=FALSE}, "Group/Flat (0:group)"=FALSE, "CollapsedNodes"=[], "Show/Hide Cols"=[], "Filtered Paths"=[], "View"=enum."Group By Library", "File Extension Filters"=[], "Filter Global VIs"=FALSE, "Shared"=refnum, "Active Filters"=refnum, "Refresh Rate (ms)"=0}, "Force Update"=FALSE}, Variant=w932) -> (data=w930:cluster{"UI State":T2, "Force Update":bool}, error out=w926:errorcluster)
            n455 = Unbundle By Name(w930) -> ("UI State"=w924:T2, "Force Update"=w928:bool)
            n456 = call "Add VIs and their Protperties to Tree.vi"("Force Tree Update (F)"=w928, "error in"=w926, "ConfigInfo in"=w924) -> ("error out"=w927:errorcluster)  [unwired: 7 in, 1 out]
            n457 = Bundle By Name(cluster=w933, "UIConfig"=w924) -> (w925:T3)
          }
          frame "UI Data Updated" {
            n458 = Unbundle By Name(w935) -> ("UIConfig"=w934:T2)
            n459 = Variant To Data(error in=w939, type=w934, Variant=w940) -> (data=w936:T2, error out=w937:errorcluster)
            n460 = Bundle By Name(cluster=w935, "UIConfig"=w936) -> (w938:T3)
          }
          frame "Exit" {
            w941 = 10000  # timeout (ms)
            n461 = Unbundle By Name(w944) -> ("Plugins"=w942:refnum<class "LVTM_Plugin.lvclass">[], "Shared"=w943:refnum<data-value>)
            n462 = Release Queue(queue=w947, error in (no error)=w945) -> (error out=w946:errorcluster)  [unwired: 1 in, 2 out]
            n463 = Delete Data Value Reference(data value reference=w943) -> ()  [unwired: 1 in, 2 out]
            n464 = for {
              tunnel: w942 -> [w951] mode=indexing
              tunnel: w941 -> [w950]
              tunnel: [w949] -> _
              n465 = call-dynamic "Shutdown.vi"("timeout in ms (-1)"=w950, "LVTM_Plugin"=w951) -> ("error out"=w949:errorcluster)  [unwired: 8 in, 1 out]
            }
          }
        }
      }
      frame True {
        # "Timed out. Check if any of the tracked VIs have changed."
        n466 = Unbundle By Name(w955) -> ("UIConfig"=w954:T2)
        n467 = call "Check for changed Items and update tree.vi"("error in"=w953, "Configuration"=w954) -> ("error out"=w952:errorcluster)  [unwired: 9 in]
      }
    }
    n468 = call "Report Error.vi"("error in"=w899) -> ("error out"=w896:errorcluster)  [unwired: 10 in]
  }
  n469 = call "Write Configuration to File.vi"(11:w10) -> ()  [unwired: 10 in, 1 out]
  n470 = Unregister For Events(event registration refnum=w24, error in=w21) -> (error out=w12:errorcluster)
  n471 = call "Request Events FG.vi"("Action (Get)"=enum16{"Initialize", "Get", "Destroy"}."Destroy" ("Action"), "error in"=w12) -> ("error out"=w13:errorcluster)  [unwired: 8 in, 1 out]
  n472 = Merge Errors(w13, w2) -> (w3:errorcluster)
  n473 = call <userlib>:"Abort Balloon Engine.vi"("error in (no error)"=w3) -> ("error out"=w19:errorcluster)  [unwired: 10 in]
  n474 = disable-structure shown="Disabled" {
    disable-tunnel: w19 -> [w956 _]
    frame Disabled {
      # "exit"
      n475 = invoke class="VI" method="FP.Close"(error in=w956) -> ()  [unwired: 2 in, 3 out]
    }
    frame Enabled {
    }
  }
